vi "lv_icon.vi"(10 "Color icon in":T2, 11 "BW icon in":T2) -> (0 "Error code out":i32=43, 2 "Color icon out":T2, 3 "BW icon out":T2)   [LabVIEW 2021, in "lv_icon.lvlib"]
doc: "<p>Display this dialog box in one of the following ways:</p>\n\n<ul>\n<li>Double-click the <a href=\"nihelplauncher://docs/csh?context=lvcore_lvconcepts_using_icons\">icon</a> in the upper right corner of the front panel window, block diagram window, or <a href=\"nihelplauncher://docs/csh?context=lvcore_lvconcepts_custom_cont_ind_type\">Control Editor</a> window.</li>\n<li>Right-click the icon in the upper right corner of the front panel window, block diagram window, or <strong>Control Editor</strong> window and select <strong>Edit Icon</strong> from the shortcut menu.</li>\n<li>Select <strong>File<span class=\"U+187\">>></span>VI Properties</strong> or <strong>File<span class=\"U+187\">>></span>Control Properties</strong> to display the <a href=\"nihelplauncher://docs/csh?context=lvcore_lvdialog_vi_properties_dialog_box\">VI Properties</a> dialog box or <strong>Control Properties</strong> dialog box, respectively. Then select <strong>General</strong> from the <strong>Category</strong> pull-down menu and click the <strong>Edit Icon</strong> button.</li>\n<li>Right-click a project library, statechart, class, or XControl item in the <a href=\"nihelplauncher://docs/csh?context=lvcore_lvconcepts_using_labview_projects\">Project Explorer</a> window and select <strong> Properties</strong> from the shortcut menu to display the corresponding <strong>Properties</strong> dialog box. Then click the <strong>Edit</strong> button on the <strong>General Settings</strong> page.</li>\n</ul>\n\n<p>Use this dialog box to <a href=\"nihelplauncher://docs/csh?context=lvcore_lvhowto_creating_icons\">create and edit icons</a>.</p>"
uses:
  <vilib>/LabVIEW Icon API/lv_icon/lv_icon.lvlib
  <vilib>/LabVIEW Icon API/lv_icon/Controls/BodyText.ctl
  <vilib>/LabVIEW Icon API/lv_icon/Controls/Font.ctl
  <vilib>/LabVIEW Icon API/lv_icon/Controls/Alignment.ctl
  <vilib>/LabVIEW Icon API/lv_icon/Controls/Layer.ctl
  <resource>/plugins/NIIconEditor/Controls/LayerList.ctl
  <resource>/plugins/NIIconEditor/Controls/NewLayer.ctl
  <resource>/plugins/NIIconEditor/Controls/DeleteLayer.ctl
  <resource>/plugins/NIIconEditor/Controls/Arrow Up.ctl
  <resource>/plugins/NIIconEditor/Controls/Arrow Down.ctl
  <resource>/plugins/NIIconEditor/Controls/Framework Templates.ctl
  <vilib>/LabVIEW Icon API/lv_icon/Controls/Graphic.ctl
  <resource>/plugins/NIIconEditor/Controls/ColorChange.ctl
  <vilib>/LabVIEW Icon API/lv_icon/Controls/IEColor.ctl
  <resource>/plugins/NIIconEditor/Controls/Rotate.ctl
  <resource>/plugins/NIIconEditor/Controls/Flip.ctl
  <resource>/plugins/NIIconEditor/Controls/Tools.ctl
  <resource>/plugins/NIIconEditor/Controls/Pen.ctl
  <resource>/plugins/NIIconEditor/Controls/Line.ctl
  <resource>/plugins/NIIconEditor/Controls/Dropper.ctl
  <resource>/plugins/NIIconEditor/Controls/Fill.ctl
  <resource>/plugins/NIIconEditor/Controls/IERect.ctl
  <resource>/plugins/NIIconEditor/Controls/FRect.ctl
  <resource>/plugins/NIIconEditor/Controls/Circle.ctl
  <resource>/plugins/NIIconEditor/Controls/FCircle.ctl
  <resource>/plugins/NIIconEditor/Controls/Rubber.ctl
  <resource>/plugins/NIIconEditor/Controls/Text.ctl
  <resource>/plugins/NIIconEditor/Controls/Selection.ctl
  <resource>/plugins/NIIconEditor/Controls/Move.ctl
  <resource>/plugins/NIIconEditor/Controls/TextMarker.ctl
  <vilib>/picture/picture.llb/imagedata.ctl
  <resource>/plugins/NIIconEditor/Controls/Refresh.ctl
  <resource>/plugins/NIIconEditor/Controls/References Cluster.ctl
  <vilib>/Utility/miscctls.llb/LVPoint32TypeDef.ctl
  <vilib>/LabVIEW Icon API/lv_icon/Controls/Pathes.ctl
  <resource>/plugins/NIIconEditor/Controls/Path&Icon.ctl
  <resource>/plugins/NIIconEditor/Class/Ants/Ants.lvclass
  <resource>/plugins/NIIconEditor/Class/FakedArray/FakedArray.lvclass
  <vilib>/LabVIEW Icon API/lv_icon/Classes/Icon/Icon.lvclass
  <resource>/plugins/NIIconEditor/Class/Icon Library/Glyph.lvclass
panel:
  out "LabVIEW Icon out":string
  in  "LabVIEW Icon in":string
  out "Terminals":picture
  out "Preview2":picture
  out "TextMarker":T1="^"
  in  "Help":bool
  in  "Cancel":bool
  in  "OK":bool
  out "XYZ":string="X: 14\nY: 31\nZ: 1"
  out "RGB":string="R: 0\nG: 0\nB: 0"
  out "Icon":picture
  out "Clipboard":picture
  in  "Tab Control":T3(tab)
  in  "refreshTemplates":T4
  out "templates path str":string
  in  "Templates":string(tree)="<All>"
  in  "Filter templates by keyword":string
  in  "Framework Templates":T5={"Scrollbar"=0, "Path & Icon 1"={"Rectangle"={"left"=0, "top"=0, "right"=32, "bottom"=32}, "Path"=path "C:/Users/tsandris/Documents/LabVIEW Data/Icon Templates/VI/Frameworks/_blank.png", "Image"=bytes[0], "Filter"="VI\\Frameworks", "FileName"="_blank"}, "Path & Icon 2"={"Rectangle"={"left"=0, "top"=0, "right"=32, "bottom"=32}, "Path"=path "C:/Users/tsandris/Documents/LabVIEW Data/Icon Templates/Library/Frameworks/_blank.png", "Image"=bytes[0], "Filter"="Library\\Frameworks", "FileName"="_blank"}, "Path & Icon 3"={"Rectangle"={"left"=0, "top"=0, "right"=0, "bottom"=0}, "Path"=path "", "Image"=bytes[0], "Filter"="", "FileName"=""}, "Path & Icon 4"={"Rectangle"={"left"=0, "top"=0, "right"=0, "bottom"=0}, "Path"=path "", "Image"=bytes[0], "Filter"="", "FileName"=""}, "Path & Icon 5"={"Rectangle"={"left"=0, "top"=0, "right"=0, "bottom"=0}, "Path"=path "", "Image"=bytes[0], "Filter"="", "FileName"=""}, "Path & Icon 6"={"Rectangle"={"left"=0, "top"=0, "right"=0, "bottom"=0}, "Path"=path "", "Image"=bytes[0], "Filter"="", "FileName"=""}, "Path & Icon 7"={"Rectangle"={"left"=0, "top"=0, "right"=0, "bottom"=0}, "Path"=path "", "Image"=bytes[0], "Filter"="", "FileName"=""}, "Path & Icon 8"={"Rectangle"={"left"=0, "top"=0, "right"=0, "bottom"=0}, "Path"=path "", "Image"=bytes[0], "Filter"="", "FileName"=""}, "Path & Icon 9"={"Rectangle"={"left"=0, "top"=0, "right"=0, "bottom"=0}, "Path"=path "", "Image"=bytes[0], "Filter"="", "FileName"=""}, "Path & Icon 10"={"Rectangle"={"left"=0, "top"=0, "right"=0, "bottom"=0}, "Path"=path "", "Image"=bytes[0], "Filter"="", "FileName"=""}, "Path & Icon 11"={"Rectangle"={"left"=0, "top"=0, "right"=0, "bottom"=0}, "Path"=path "", "Image"=bytes[0], "Filter"="", "FileName"=""}, "Path & Icon 12"={"Rectangle"={"left"=0, "top"=0, "right"=0, "bottom"=0}, "Path"=path "", "Image"=bytes[0], "Filter"="", "FileName"=""}, "Path & Icon 13"={"Rectangle"={"left"=0, "top"=0, "right"=0, "bottom"=0}, "Path"=path "", "Image"=bytes[0], "Filter"="", "FileName"=""}, "Path & Icon 14"={"Rectangle"={"left"=0, "top"=0, "right"=0, "bottom"=0}, "Path"=path "", "Image"=bytes[0], "Filter"="", "FileName"=""}, "Path & Icon 15"={"Rectangle"={"left"=0, "top"=0, "right"=0, "bottom"=0}, "Path"=path "", "Image"=bytes[0], "Filter"="", "FileName"=""}, "Path & Icon 16"={"Rectangle"={"left"=0, "top"=0, "right"=0, "bottom"=0}, "Path"=path "", "Image"=bytes[0], "Filter"="", "FileName"=""}, "Path & Icon 17"={"Rectangle"={"left"=0, "top"=0, "right"=0, "bottom"=0}, "Path"=path "", "Image"=bytes[0], "Filter"="", "FileName"=""}, "Path & Icon 18"={"Rectangle"={"left"=0, "top"=0, "right"=0, "bottom"=0}, "Path"=path "", "Image"=bytes[0], "Filter"="", "FileName"=""}, "Path & Icon 19"={"Rectangle"={"left"=0, "top"=0, "right"=0, "bottom"=0}, "Path"=path "", "Image"=bytes[0], "Filter"="", "FileName"=""}, "Path & Icon 20"={"Rectangle"={"left"=0, "top"=0, "right"=0, "bottom"=0}, "Path"=path "", "Image"=bytes[0], "Filter"="", "FileName"=""}, "Path & Icon 21"={"Rectangle"={"left"=0, "top"=0, "right"=0, "bottom"=0}, "Path"=path "", "Image"=bytes[0], "Filter"="", "FileName"=""}, "Path & Icon 22"={"Rectangle"={"left"=0, "top"=0, "right"=0, "bottom"=0}, "Path"=path "", "Image"=bytes[0], "Filter"="", "FileName"=""}, "Path & Icon 23"={"Rectangle"={"left"=0, "top"=0, "right"=0, "bottom"=0}, "Path"=path "", "Image"=bytes[0], "Filter"="", "FileName"=""}, "Path & Icon 24"={"Rectangle"={"left"=0, "top"=0, "right"=0, "bottom"=0}, "Path"=path "", "Image"=bytes[0], "Filter"="", "FileName"=""}, "Path & Icon 25"={"Rectangle"={"left"=0, "top"=0, "right"=0, "bottom"=0}, "Path"=path "", "Image"=bytes[0], "Filter"="", "FileName"=""}, "Path & Icon 26"={"Rectangle"={"left"=0, "top"=0, "right"=0, "bottom"=0}, "Path"=path "", "Image"=bytes[0], "Filter"="", "FileName"=""}, "Path & Icon 27"={"Rectangle"={"left"=0, "top"=0, "right"=0, "bottom"=0}, "Path"=path "", "Image"=bytes[0], "Filter"="", "FileName"=""}, "Path & Icon 28"={"Rectangle"={"left"=0, "top"=0, "right"=0, "bottom"=0}, "Path"=path "", "Image"=bytes[0], "Filter"="", "FileName"=""}, "Path & Icon 29"={"Rectangle"={"left"=0, "top"=0, "right"=0, "bottom"=0}, "Path"=path "", "Image"=bytes[0], "Filter"="", "FileName"=""}, "Path & Icon 30"={"Rectangle"={"left"=0, "top"=0, "right"=0, "bottom"=0}, "Path"=path "", "Image"=bytes[0], "Filter"="", "FileName"=""}}
  in  "Body Text":T7={"Line 1 text"="", "Line 2 text"="", "Line 3 text"="", "Line 4 text"="", "Line 1 color"=0, "Line 2 color"=0, "Line 3 color"=0, "Line 4 color"=0, "Body Text Spec"={"Font"="", "Alignment"=1, "Size"=9}, "Center text vertically"=TRUE, "Capitalize Text"=TRUE} {"Body Text Spec"."Alignment" items=["left", "center", "right"]}
  in  "Filter glyphs by keyword":string
  in  "Glyphs":string(tree)="<All>"
  out "glyph path str":string
  out "Glyphs []":T6[][](array[typedef])
  in  "refreshGlyphs":T4
  in  "Add Layer":T10
  in  "Remove Layer":T11
  in  "Move Down":T12
  in  "Move Up":T13
  in  "Icon Template":T14={"LayerIcon"=bytes[0], "LayerName"="", "Opacity"=100, "Visibility?"=TRUE} {"Opacity" scale=0.0..100.0}
  in  "Icon Text":T14={"LayerIcon"=bytes[0], "LayerName"="Icon Text", "Opacity"=100, "Visibility?"=TRUE} {"Opacity" scale=0.0..100.0}
  in  "User Layers":T15={"Scrollbar"=0, "Layer 1"={"LayerIcon"=bytes[0], "LayerName"="VI Icon", "Opacity"=100, "Visibility?"=TRUE}, "Layer 2"={"LayerIcon"=bytes[3230], "LayerName"="", "Opacity"=100, "Visibility?"=TRUE}, "Layer 3"={"LayerIcon"=bytes[3230], "LayerName"="", "Opacity"=100, "Visibility?"=TRUE}, "Layer 4"={"LayerIcon"=bytes[3230], "LayerName"="", "Opacity"=100, "Visibility?"=TRUE}} {"Layer 4"."Opacity" scale=0.0..100.0; "Layer 3"."Opacity" scale=0.0..100.0; "Layer 2"."Opacity" scale=0.0..100.0; "Layer 1"."Opacity" scale=0.0..100.0}
  out "Preview":picture
  in  "Horizontal Flip":T16
  in  "Clockwise Rotate":T17
  in  "Swap":T18
  in  "Line Color":T19
  in  "Fill Color":T19=16777215
  in  "Tools":T20=enum."Rectangle"
  # "Clipboard control. Anything made on this\ncontrol will show up in the clipboard image data."
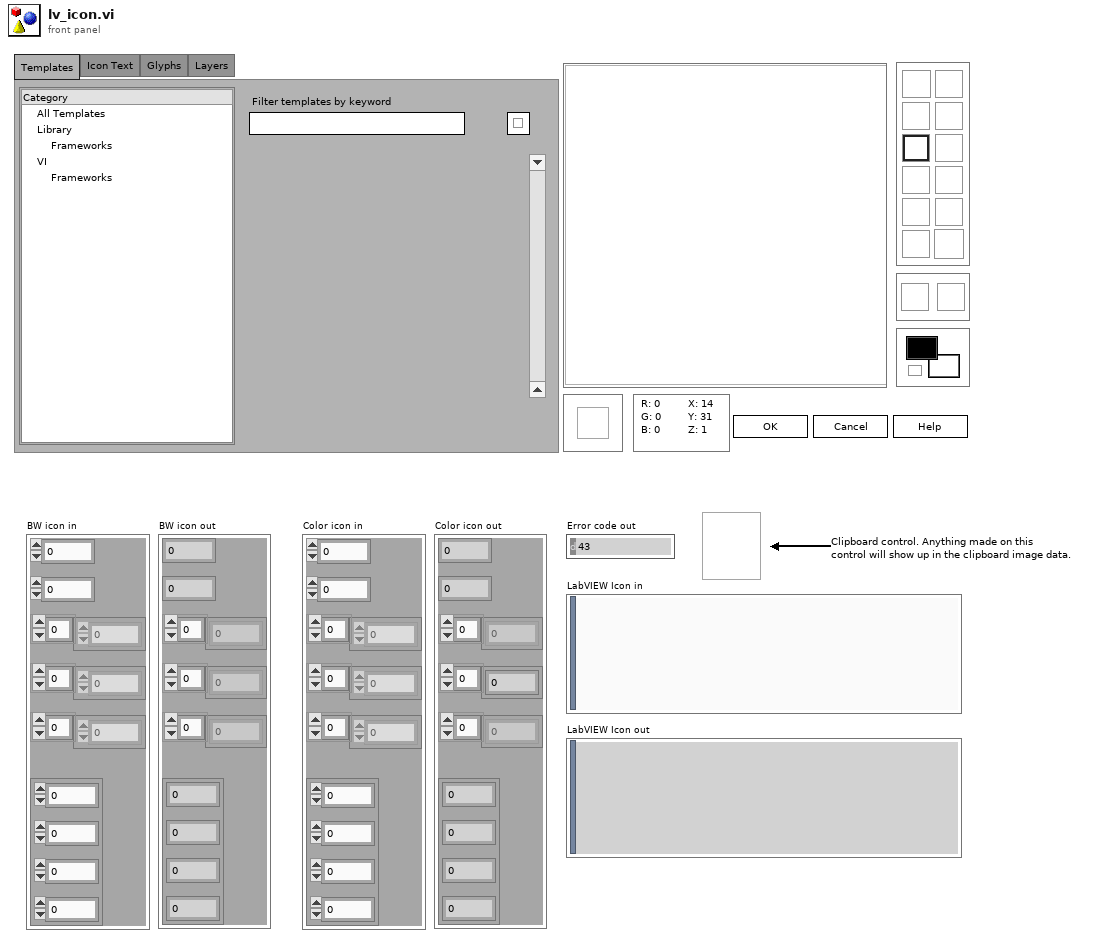
[diagram p1: front panel]
types:
  T1 = typedef "TextMarker.ctl" = string
  T2 = typedef "imagedata.ctl" = cluster{"image type":i32, "image depth":i32, "image":u8[], "mask":u8[], "colors":u32[], "Rectangle":cluster{"left":i16, "top":i16, "right":i16, "bottom":i16}}
  T3 = enum32{"Templates", "Icon Text", "Glyphs", "Layers"}
  T4 = typedef "Refresh.ctl" = bool
  T5 = typedef "Framework Templates.ctl" = cluster{"Scrollbar":i32, "Path & Icon 1":T6, "Path & Icon 2":T6, "Path & Icon 3":T6, "Path & Icon 4":T6, "Path & Icon 5":T6, "Path & Icon 6":T6, "Path & Icon 7":T6, "Path & Icon 8":T6, "Path & Icon 9":T6, "Path & Icon 10":T6, "Path & Icon 11":T6, "Path & Icon 12":T6, "Path & Icon 13":T6, "Path & Icon 14":T6, "Path & Icon 15":T6, "Path & Icon 16":T6, "Path & Icon 17":T6, "Path & Icon 18":T6, "Path & Icon 19":T6, "Path & Icon 20":T6, "Path & Icon 21":T6, "Path & Icon 22":T6, "Path & Icon 23":T6, "Path & Icon 24":T6, "Path & Icon 25":T6, "Path & Icon 26":T6, "Path & Icon 27":T6, "Path & Icon 28":T6, "Path & Icon 29":T6, "Path & Icon 30":T6}
  T6 = typedef "Graphic.ctl" = cluster{"Rectangle":cluster{"left":i16, "top":i16, "right":i16, "bottom":i16}, "Path":path, "Image":picture, "Filter":string, "FileName":string}
  T7 = typedef "BodyText.ctl" = cluster{"Line 1 text":string, "Line 2 text":string, "Line 3 text":string, "Line 4 text":string, "Line 1 color":u32, "Line 2 color":u32, "Line 3 color":u32, "Line 4 color":u32, "Body Text Spec":cluster{"Font":T8, "Alignment":T9, "Size":u8}, "Center text vertically":bool, "Capitalize Text":bool}
  T8 = typedef "Font.ctl" = string
  T9 = typedef "Alignment.ctl" = u16
  T10 = typedef "NewLayer.ctl" = bool
  T11 = typedef "DeleteLayer.ctl" = bool
  T12 = typedef "Arrow Down.ctl" = bool
  T13 = typedef "Arrow Up.ctl" = bool
  T14 = typedef "Layer.ctl" = cluster{"LayerIcon":picture, "LayerName":string, "Opacity":u8, "Visibility?":bool}
  T15 = typedef "LayerList.ctl" = cluster{"Scrollbar":i32, "Layer 1":T14, "Layer 2":T14, "Layer 3":T14, "Layer 4":T14}
  T16 = typedef "Flip.ctl" = bool
  T17 = typedef "Rotate.ctl" = bool
  T18 = typedef "ColorChange.ctl" = bool
  T19 = typedef "IEColor.ctl" = u32
  T20 = typedef "Tools.ctl" = enum32{"Pencil", "Line", "Dropper", "Fill", "Rectangle", "Filled Rectangle", "Ellipse", "Filled Ellipse", "Eraser", "Text", "Select", "Move"}
  T21 = enum32{"Invalid", "Standard", "Closed", "Hidden", "Minimized", "Maximized"}
  T22 = typedef "lv_icon.lvlib/References Cluster.ctl" = cluster{"Add Layer":refnum<vi>, "Remove Layer":refnum<vi>, "Line Text":refnum<vi>[], "Body Text Spec":refnum<vi>, "DNL_Font":refnum<vi>, "glyph path str":refnum<vi>, "templates path str":refnum<vi>, "Arrow Up":refnum<vi>, "Arrow Down":refnum<vi>, "IE VI Ref":refnum<vi>, "Glyphs tree":refnum<vi>, "Templates tree":refnum<vi>, "Layer Icon Text":refnum<vi>, "Layer Template":refnum<vi>, "Body Text":refnum<vi>, "Search Templates":refnum<vi>, "TextMarker":refnum<vi>, "Tab Control":refnum<vi>, "Search Glyphs":refnum<vi>, "Line Color":refnum<vi>, "DNL_Glyphs []":refnum<vi>, "Fill Color":refnum<vi>, "Tools":refnum<vi>, "Icon":refnum<vi>, "Preview":refnum<vi>, "Ants":refnum<vi>, "Terminals":refnum<vi>, "menu reference":refnum<k9>, "LayerNames":refnum<vi>[], "GlyphLoadAnimation":refnum<vi>, "TemplateLoadAnimation":refnum<vi>, "refreshGlyphs":refnum<vi>, "refreshTemplates":refnum<vi>}
  T23 = cluster{"Global stop?":refnum<user-event>, "Templates":refnum<user-event>, "Glyphs":refnum<user-event>}
  T24 = typedef "lv_icon.lvlib/Global Data.ctl" = cluster{"Class":T25, "Ref":T22, "Support":T26}
  T25 = typedef "IE Classes.ctl" = cluster{"Ants":refnum<class "Ants.lvclass">, "Layer":refnum<class "FakedArray.lvclass">, "Templates":refnum<class "FakedArray.lvclass">, "Icon":refnum<class "Icon.lvclass">, "Glyph":refnum<class "Glyph.lvclass">, "Settings":refnum<class "Settings.lvclass">, "Tools":refnum<class "Tools Paint.lvclass">}
  T26 = typedef "SupportClass.ctl" = cluster{"AntsRect":cluster{"left":i16, "top":i16, "right":i16, "bottom":i16}, "Mouse Move Coords":T27, "Mouse Down Coords":T27, "Temp Coord":T27, "Action":T28, "Edge Color":T19, "Fill Color":T19, "Mouse Down?":bool, "Draft Mode?":bool, "Temp Icon":picture, "CTRL Pressed":bool, "Move Selection?":bool, "AntsRect Orig":cluster{"left":i16, "top":i16, "right":i16, "bottom":i16}, "Text":string, "TM Set?":bool, "Mouse inside icon?":bool, "Tool (old value)":u32, "Pencil Move Color":u32, "Swap Colors?":bool, "Shift pressed?":bool}
  T27 = typedef "LVPoint32TypeDef.ctl" = cluster{"Horizontal":i32, "Vertical":i32}
  T28 = typedef "SupportClass_Action.ctl" = enum16{"Default", "Move Selection", "Glyph Library", "Tool"}
  T29 = typedef "Pathes.ctl" = enum16{"Root Path", "Icon Templates", "Icon Templates VI", "Icon Templates Lib", "Glyphs"}
  T30 = typedef "Path&Icon.ctl" = cluster{"Rectangle":cluster{"left":i16, "top":i16, "right":i16, "bottom":i16}, "Path":path, "Image":picture, "Filter":string, "FileName":string}
  T31 = typedef "lveventtype.ctl" = enum32{"Null", "Timeout", "Annotation Menu Selection", "Annotation Menu Selection?", "App Instance Close", "App Instance Close?", "Autoscale Range Change", "Bookmark Info Change", "Cell Edit", "Cell Edit?", "Cursor Grab", "Cursor Grab?", "Cursor Menu Selection", "Cursor Menu Selection?", "Cursor Move", "Cursor Release", "Data Change", "Direction Change", "Display State Change", "Drag Ended", "Drag Enter", "Drag Leave", "Drag Over", "Drag Source Update", "Drag Starting", "Drag Starting?", "Drop", "Exec State Change", "Key Down", "Key Down?", "Key Repeat", "Key Repeat?", "Key Up", "Listbox Double Click", "Menu Activation?", "Menu Selection (App)", "Menu Selection? (App)", "Menu Selection (User)", "Mouse Down", "Mouse Down?", "Mouse Enter", "Mouse Leave", "Mouse Move", "Mouse Up", "Mouse Wheel", "NI Security User Change (App)", "Pane Size", "Panel Close", "Panel Close?", "Panel Resize", "Plot Attribute Change", "Scale Range Change", "Shortcut Menu Activation?", "Shortcut Menu Selection (App)", "Shortcut Menu Selection? (App)", "Shortcut Menu Selection (User)", "Tree Double Click", "Tree Drag", "Tree Drag?", "Tree Drop", "Tree Drop?", "Tree Item Close", "Tree Item Close?", "Tree Item Open", "Tree Item Open?", "User Event", "Value Change"}
  T32 = typedef "eventvkey.ctl" = enum16{"ASCII", "Enter", "Return", "Shift", "Ctrl", "Alt", "Cmd", "Opt", "Caps", "NumLock", "Clear", "Break", "Up", "Down", "Left", "Right", "Insert", "Delete", "Home", "End", "PageUp", "PageDown", "Escape", "Help", "Pause", "ScrollLock", "F1", "F2", "F3", "F4", "F5", "F6", "F7", "F8", "F9", "F10", "F11", "F12", "F13", "F14", "F15", "F16", "F17", "F18", "F19", "F20", "F21", "F22", "F23", "F24", "Play", "VolumeUp", "VolumeDown", "Mute", "Two Byte Char"}
  T33 = cluster{"Shift":bool, "Ctrl":bool, "Alt":bool, "Cmd":bool, "Opt":bool}
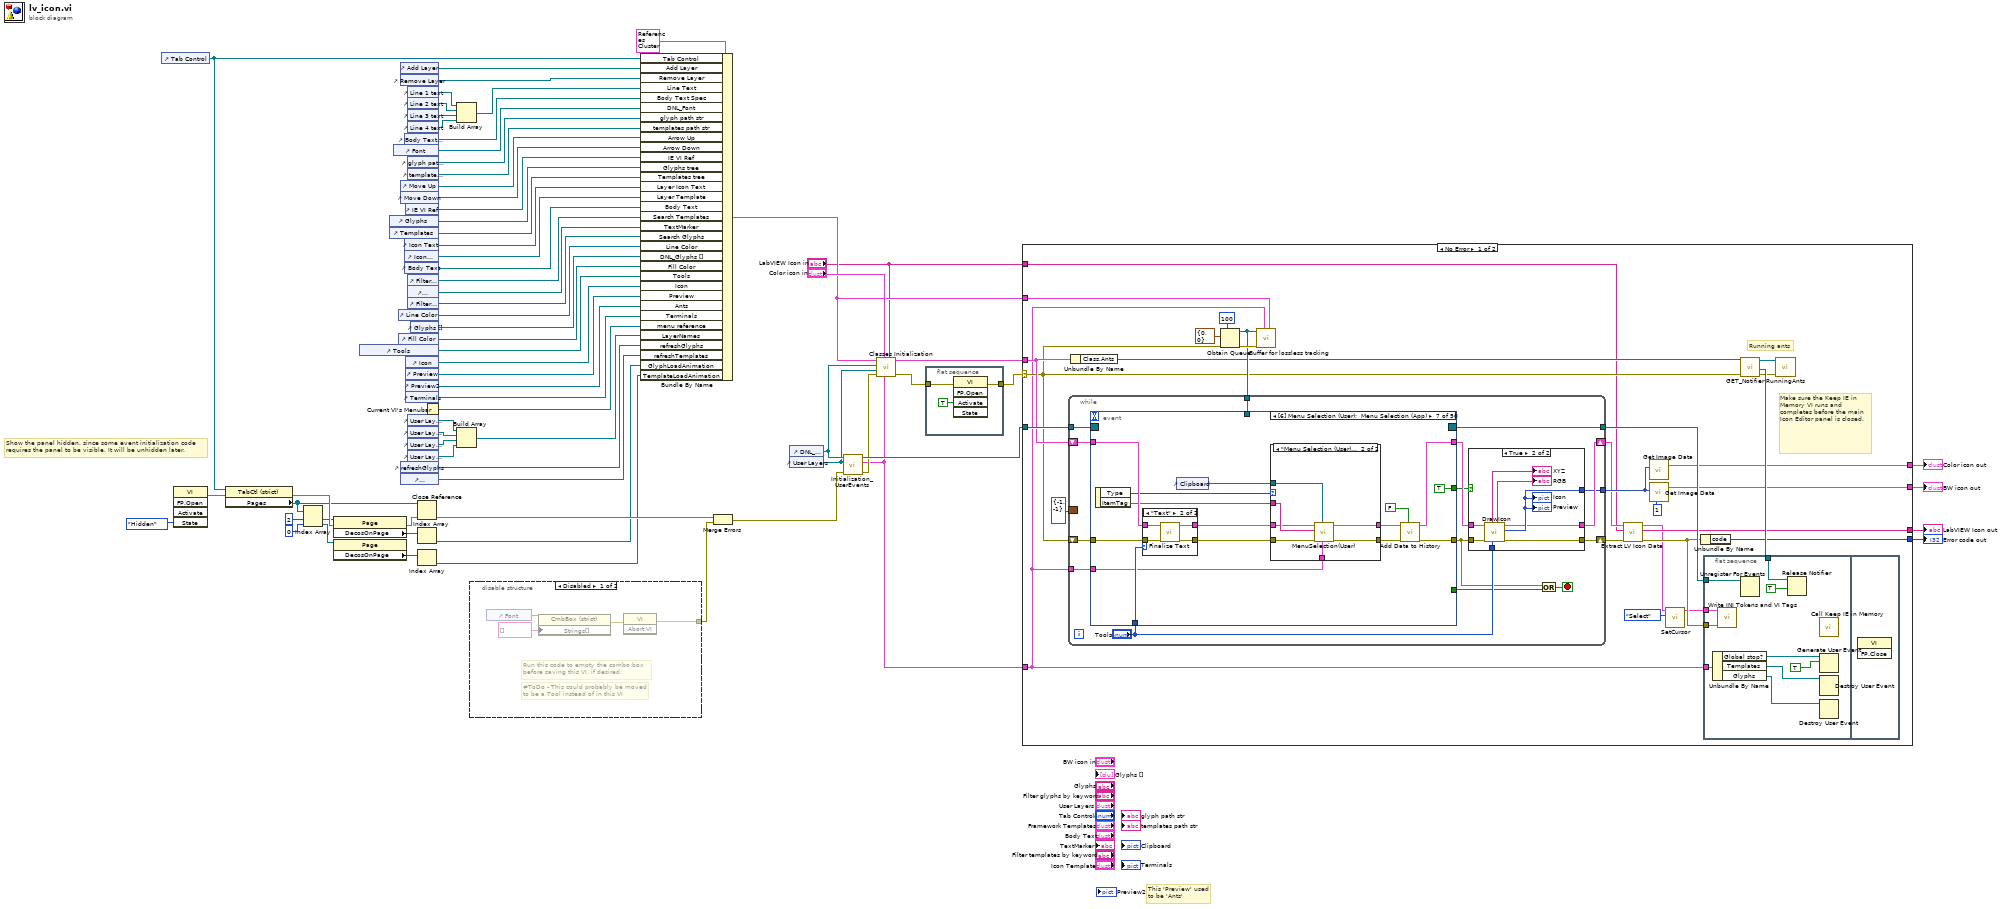
[diagram p0: block diagram]
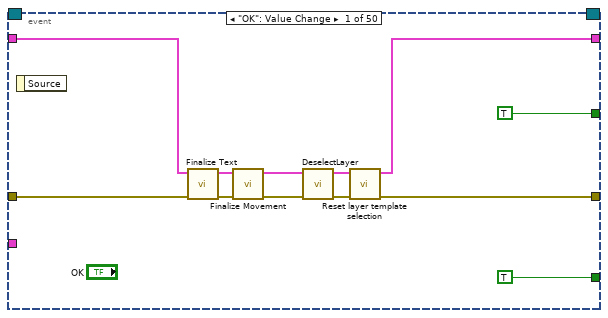
[diagram p4: hidden frame]
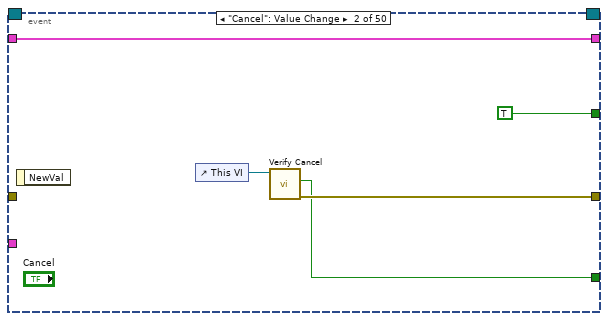
[diagram p5: hidden frame]
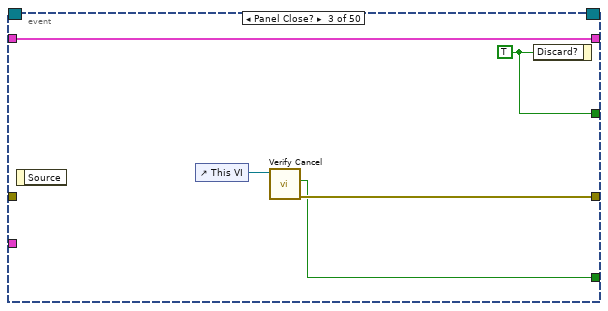
[diagram p6: hidden frame]
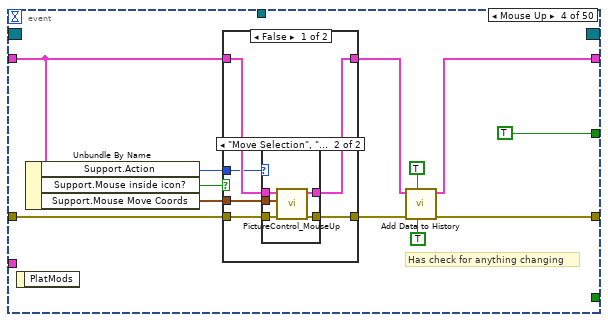
[diagram p7: hidden frame]
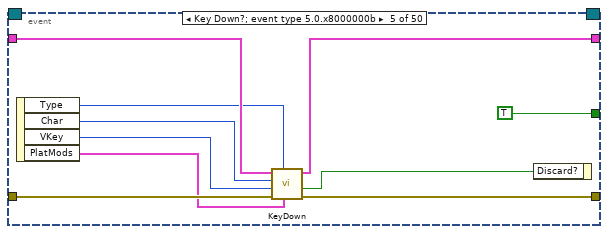
[diagram p10: hidden frame]
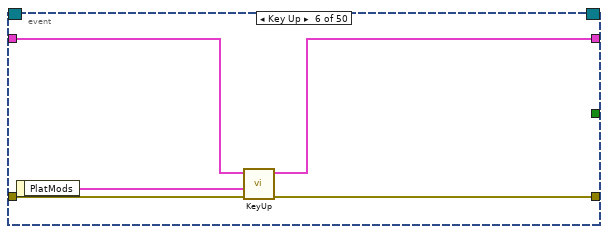
[diagram p11: hidden frame]
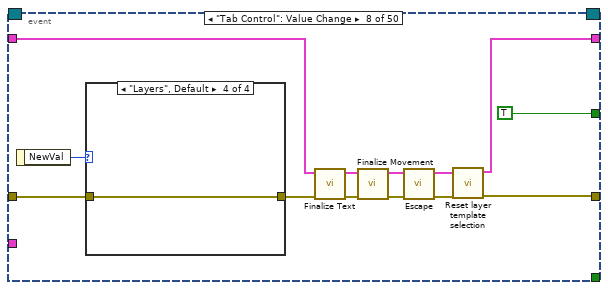
[diagram p14: hidden frame]
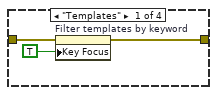
[diagram p15: hidden frame]
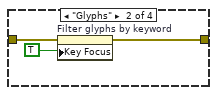
[diagram p16: hidden frame]
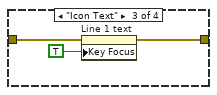
[diagram p17: hidden frame]
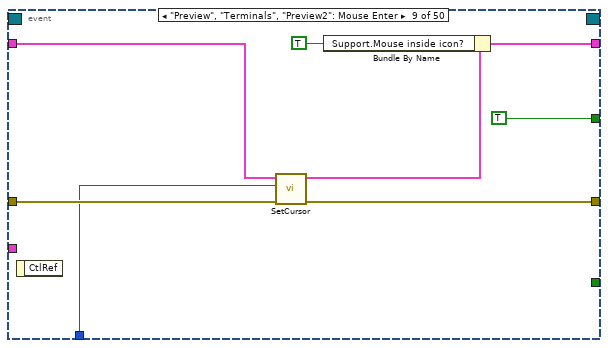
[diagram p18: hidden frame]
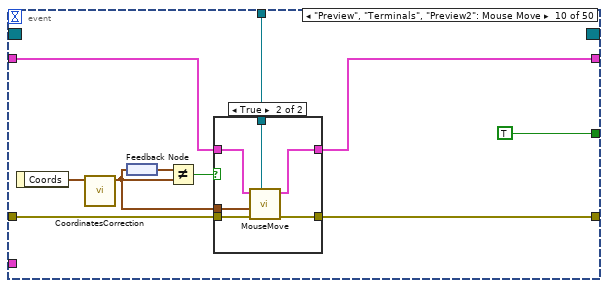
[diagram p19: hidden frame]
diagram:
  # "Show the panel hidden, since some event initialization code requires the panel to be visible. It will be unhidden later."
  # "This 'Preview' used\nto be 'Ants'"
  n1 = control-ref of="Tab Control"() -> (w4:refnum<vi>)
  n2 = invoke class="VI" method="FP.Open"("State"=T21."Hidden") -> (error out=w1:errorcluster)  [unwired: 4 in, 4 out]
  n3 = property class="TabCtl (strict)"(reference=w4, error in=w1) -> (error out=w14:errorcluster, "Pages"=w6:refnum<vi>[])  [unwired: 1 out]
  n4 = Index Array(array=w6, index #1=2 ("index"), index #2=0 ("index")) -> (element #1=w10:refnum<vi>, element #2=w11:refnum<vi>)
  n5 = property class="Page"(reference=w10, error in=w14) -> (error out=w7:errorcluster, "DecosOnPage"=w9:refnum<vi>[])  [unwired: 1 out]
  n6 = property class="Page"(reference=w11) -> ("DecosOnPage"=w8:refnum<vi>[])  [unwired: 1 in, 2 out]
  n7 = control-ref of="Tools"() -> (w68:refnum<vi>)
  n8 = control-ref of="Glyphs"() -> (w52:refnum<vi>)
  n9 = control-ref of="Templates"() -> (w53:refnum<vi>)
  n10 = control-ref of="Font"() -> (w34:refnum<vi>)
  n11 = control-ref of="Line Color"() -> (w66:refnum<vi>)
  n12 = control-ref of="Fill Color"() -> (w67:refnum<vi>)
  n13 = control-ref of="Add Layer"() -> (w37:refnum<vi>)
  n14 = control-ref of="Remove Layer"() -> (w38:refnum<vi>)
  n15 = control-ref of="Move Up"() -> (w49:refnum<vi>)
  n16 = control-ref of="Move Down"() -> (w50:refnum<vi>)
  n17 = control-ref of="refreshGlyphs"() -> (w24:refnum<vi>)
  n18 = control-ref of="refreshTemplates"() -> (w25:refnum<vi>)
  n19 = control-ref of="Body Text Spec"() -> (w46:refnum<vi>)
  n20 = control-ref of="Icon Text"() -> (w55:refnum<vi>)
  n21 = control-ref of="Icon Template"() -> (w56:refnum<vi>)
  n22 = control-ref of="Body Text"() -> (w61:refnum<vi>)
  n23 = control-ref of="IE VI Ref"() -> (w51:refnum<vi>)
  n24 = control-ref of="Icon"() -> (w69:refnum<vi>)
  n25 = control-ref of="Preview"() -> (w70:refnum<vi>)
  n26 = control-ref of="Preview2"() -> (w45:refnum<vi>)
  n27 = control-ref of="Terminals"() -> (w60:refnum<vi>)
  n28 = control-ref of="Line 1 text"() -> (w40:refnum<vi>)
  n29 = control-ref of="Line 2 text"() -> (w41:refnum<vi>)
  n30 = control-ref of="Line 3 text"() -> (w42:refnum<vi>)
  n31 = control-ref of="Line 4 text"() -> (w43:refnum<vi>)
  n32 = control-ref of="glyph path str"() -> (w47:refnum<vi>)
  n33 = control-ref of="templates path str"() -> (w48:refnum<vi>)
  n34 = control-ref of="Filter templates by keyword"() -> (w63:refnum<vi>)
  n35 = control-ref of="TextMarker"() -> (w64:refnum<vi>)
  n36 = control-ref of="Filter glyphs by keyword"() -> (w65:refnum<vi>)
  n37 = control-ref of="User Layer 1"() -> (w29:refnum<vi>)
  n38 = control-ref of="User Layer 2"() -> (w30:refnum<vi>)
  n39 = control-ref of="User Layer 3"() -> (w31:refnum<vi>)
  n40 = control-ref of="User Layer 4"() -> (w32:refnum<vi>)
  n41 = control-ref of="Glyphs []"() -> (w35:refnum<vi>)
  n42 = Close Reference(reference=w6, error in (no error)=w7) -> (error out=w5:errorcluster)
  n43 = Index Array(array=w9) -> (element=w3:refnum<vi>)  [unwired: 1 in]
  n44 = Index Array(array=w8) -> (element=w2:refnum<vi>)  [unwired: 1 in]
  n45 = Current VI's Menubar() -> (w59:refnum<k9>)
  n46 = Build Array(w40, w41, w42, w43) -> (w39:refnum<vi>[])
  n47 = Build Array(w29, w30, w31, w32) -> (w27:refnum<vi>[])
  n48 = disable-structure shown="Disabled" {
    disable-tunnel: [w72 _] -> w16
    frame Disabled {
      # "#ToDo - This could probably be moved\nto be a Tool instead of in this VI"
      # "Run this code to empty the combo box\nbefore saving this VI, if desired."
      n49 = control-ref of="Font"() -> (w75:refnum<vi>)
      n50 = property class="CmbBox (strict)"(reference=w75, "Strings[]"=string[] [] ("Strings []")) -> (error out=w73:errorcluster)  [unwired: 1 in, 1 out]
      n51 = invoke class="VI" method="Abort VI"(error in=w73) -> (error out=w72:errorcluster)  [unwired: 2 in, 2 out]
    }
    frame Enabled {
    }
  }
  n52 = Bundle By Name(cluster=T22 {"Add Layer"=refnum, "Remove Layer"=refnum, "Line Text"=[], "Body Text Spec"=refnum, "DNL_Font"=refnum, "glyph path str"=refnum, "templates path str"=refnum, "Arrow Up"=refnum, "Arrow Down"=refnum, "IE VI Ref"=refnum, "Glyphs tree"=refnum, "Templates tree"=refnum, "Layer Icon Text"=refnum, "Layer Template"=refnum, "Body Text"=refnum, "Search Templates"=refnum, "TextMarker"=refnum, "Tab Control"=refnum, "Search Glyphs"=refnum, "Line Color"=refnum, "DNL_Glyphs []"=refnum, "Fill Color"=refnum, "Tools"=refnum, "Icon"=refnum, "Preview"=refnum, "Ants"=refnum, "Terminals"=refnum, "menu reference"=refnum, "LayerNames"=[], "GlyphLoadAnimation"=refnum, "TemplateLoadAnimation"=refnum, "refreshGlyphs"=refnum, "refreshTemplates"=refnum} ("references"), "Tab Control"=w4, "Add Layer"=w37, "Remove Layer"=w38, "Line Text"=w39, "Body Text Spec"=w46, "DNL_Font"=w34, "glyph path str"=w47, "templates path str"=w48, "Arrow Up"=w49, "Arrow Down"=w50, "IE VI Ref"=w51, "Glyphs tree"=w52, "Templates tree"=w53, "Layer Icon Text"=w55, "Layer Template"=w56, "Body Text"=w61, "Search Templates"=w63, "TextMarker"=w64, "Search Glyphs"=w65, "Line Color"=w66, "DNL_Glyphs []"=w35, "Fill Color"=w67, "Tools"=w68, "Icon"=w69, "Preview"=w70, "Ants"=w45, "Terminals"=w60, "menu reference"=w59, "LayerNames"=w27, "refreshGlyphs"=w24, "refreshTemplates"=w25, "GlyphLoadAnimation"=w3, "TemplateLoadAnimation"=w2) -> (w28:T22)
  n53 = Merge Errors(w5, w16) -> (w15:errorcluster)
  n54 = control-ref of="DNL_Framework Templates"() -> (w18:refnum<vi>)
  n55 = control-ref of="User Layers"() -> (w17:refnum<vi>)
  n56 = call <resource>:"Initialization_UserEvents.vi"("error in"=w15, "Layer Clusters"=w17, "DNL_Framework Templates"=w18) -> ("error out"=w57:errorcluster, "User events"=w19:T23, "Events"=w62:refnum<event-registration>)  [unwired: 6 out]
  n57 = call <resource>:"Classes Initialization.vi"("LabVIEW Icon in"="LabVIEW Icon in", "User events"=w19, "Color icon in"="Color icon in", "error in"=w57, "Layer Clusters"=w17, "DNL_Framework Templates"=w18, "Ref Cluster"=w28) -> ("error out"=w21:errorcluster, "Data out"=w44:T24)  [unwired: 3 out]
  n58 = flat-sequence {
    tunnel: w21 -> [w77]
    tunnel: [w76] -> w20
    frame #0 {
      n59 = invoke class="VI" method="FP.Open"(error in=w77, "Activate"=TRUE ("Activate?")) -> (error out=w76:errorcluster)  [unwired: 3 in, 4 out]
    }
  }
  n60 = case shown="No Error" w20 {
    selector: w20 -> [w88 w777]
    tunnel: w62 -> [w105 _]
    tunnel: [w103 w778] -> w58
    tunnel: [w100 _] -> w54
    tunnel: w19 -> [w79 _]
    tunnel: w44 -> [w93 _]
    tunnel: w28 -> [w91 _]
    tunnel: [w90 _] -> w36
    tunnel: "LabVIEW Icon in" -> [w83 w776]
    tunnel: [w86 w776] -> w33
    frame No Error {
      # "Make sure the Keep IE in Memory VI runs and completes before the main Icon Editor panel is closed."
      # "Running ants"
      n61 = Unbundle By Name(w93) -> ("Class.Ants"=w92:refnum<class "Ants.lvclass">)
      n62 = Obtain Queue(max queue size (-1, unlimited)=100, element data type=T27 {"Horizontal"=0, "Vertical"=0} ("Coords"), error in (no error)=w88) -> (queue out=w94:refnum<queue>, error out=w95:errorcluster)  [unwired: 1 in, 2 out]
      n63 = while {
        shift-right: [w111] -> w85
        shift-left: w88 -> [w118]
        tunnel: [w115] -> w106
        tunnel: w105 -> [w114]
        tunnel: [w113] -> w102
        tunnel: w94 -> [w109]
        shift-right: [w120] -> w87
        shift-left: w93 -> [w108]
        border: T27 {"Horizontal"=-1, "Vertical"=-1} ("Corrected Out") -> [_]
        tunnel: w79 -> [w107]
        stop <- w116 stop-if-true
        n64 = event shown="[6] Menu Selection (User);  Menu Selection (App)" {
          selector: w114 -> [_ _ _ _ _ _ _ _ _ _ _ _ _ _ _ _ _ _ _ _ _ _ _ _ _ _ _ _ _ _ _ _ _ _ _ _ _ _ _ _ _ _ _ _ _ _ _ _ _ _]
          dyn-events: [_ _ _ _ _ _ _ _ _ _ _ _ _ _ _ _ _ _ _ _ _ _ _ _ _ _ _ _ _ _ _ _ _ _ _ _ _ _ _ _ _ _ _ _ _ _ _ _ _ _] -> w115
          timeout: _ -> [_ _ _ _ _ _ _ _ _ _ _ _ _ _ _ _ _ _ _ _ _ _ _ _ _ _ _ _ _ _ _ _ _ _ _ _ _ _ _ _ _ _ _ _ _ _ _ _ _ _]
          tunnel: [w137 w147 w152 w157 w189 w195 w199 w234 w255 w265 w278 w295 w299 w305 w309 w322 w334 w348 w363 w374 w399 w406 w417 w433 w454 w462 w480 w500 w505 w509 w516 w527 w547 w562 w577 w588 w601 w617 w626 w635 w658 w671 w686 w696 w698 w717 w734 w754 w761 w763] -> w112
          tunnel: w118 -> [w139 _ _ w163 w190 w194 w207 w236 w256 w266 w278 w296 w302 w307 w314 w326 w333 w342 w365 w383 w400 w409 w422 w435 w457 w476 w488 w501 w506 w510 w517 w539 w552 w565 w581 w589 w607 w621 w627 w638 w661 w679 w689 w695 w707 w724 w738 w755 w761 w764]
          tunnel: [TRUE w146 w151 _ _ _ _ _ _ _ _ _ _ _ _ _ _ _ _ _ _ _ _ _ _ _ _ _ _ _ _ _ _ _ _ _ _ _ _ _ _ _ _ _ _ _ _ _ _ _] -> w117
          tunnel: "Tools" -> [_ _ _ _ _ _ w205 _ w254 _ _ _ _ _ _ _ _ _ _ _ _ _ _ _ _ _ _ _ _ _ _ _ _ _ _ _ _ _ _ _ _ _ _ _ _ _ _ _ _ _]
          tunnel: [TRUE TRUE ("Yes") w150 TRUE ("Yes") TRUE _ TRUE TRUE TRUE TRUE _ TRUE TRUE _ TRUE TRUE TRUE TRUE TRUE TRUE _ _ TRUE TRUE _ _ _ _ _ _ TRUE TRUE TRUE _ TRUE _ TRUE _ _ TRUE TRUE _ _ _ _ _ TRUE _ _ _] -> w110
          tunnel: w109 -> [_ _ _ _ _ _ _ _ _ w263 _ _ _ _ _ _ _ _ _ _ _ _ _ _ _ _ _ _ _ _ _ _ _ _ _ _ _ _ _ _ _ _ _ _ _ _ _ _ _ _]
          tunnel: w108 -> [w136 w148 w153 w162 w185 w193 w210 w232 w252 w262 w275 w292 w298 w304 w313 w325 w332 w344 w358 w370 w403 w405 w413 w431 w450 w467 w485 w498 w508 w512 w514 w535 w543 w560 w573 w586 w599 w623 w624 w645 w656 w669 w685 w693 w703 w722 w731 w752 w760 w765]
          tunnel: [w132 w148 w153 w155 w182 w191 w201 w226 w250 w261 w277 w291 w297 w303 w318 w320 w330 w347 w359 w375 w388 w404 w411 w429 w449 w460 w481 w498 w508 w511 w513 w528 w541 w559 w572 w585 w598 w615 w625 w631 w655 w673 w684 w691 w699 w716 w728 w752 w760 w765] -> w121
          tunnel: w107 -> [_ _ _ _ _ _ w197 _ _ _ _ _ _ _ _ _ _ _ _ _ _ _ _ _ _ _ _ w499 _ _ _ _ _ _ _ _ _ _ _ _ _ _ _ _ _ _ _ w753 _ _]
          event "OK": Value Change {
            n65 = event-data() -> ()  [unwired: 2 out]
            n66 = call <resource>:"Finalize Text.vi"("error in (no error)"=w139, "Data in"=w136) -> ("error out"=w140:errorcluster, "Data out"=w135:T24)  [unwired: 8 out]
            n67 = call <resource>:"Finalize Movement.vi"("error in (no error)"=w140, "Data in"=w135) -> ("error out"=w141:errorcluster, "Data out"=w134:T24)  [unwired: 1 in, 7 out]
            n68 = call <resource>:"DeselectLayer.vi"("error in (no error)"=w141, "Data in"=w134) -> ("error out"=w138:errorcluster, "Data out"=w133:T24)  [unwired: 8 out]
            n69 = call <resource>:"Reset layer template selection.vi"("error in (no error)"=w138, "Data in"=w133) -> ("error out"=w137:errorcluster, "Data out"=w132:T24)  [unwired: 1 in, 7 out]
          }
          event "Cancel": Value Change {
            n70 = event-data() -> ()  [unwired: 2 out]
            n71 = control-ref of="This VI"() -> (w144:refnum<vi>)
            n72 = call <resource>:"Verify Cancel.vi"("Calling VI"=w144) -> ("error out"=w147:errorcluster, "Close IE"=w146:bool)  [unwired: 9 in]
          }
          event Panel Close? {
            w150 = TRUE ("Discard?")
            n73 = event-data() -> ()  [unwired: 2 out]
            n74 = control-ref of="This VI"() -> (w149:refnum<vi>)
            n75 = call <resource>:"Verify Cancel.vi"("Calling VI"=w149) -> ("error out"=w152:errorcluster, "Close IE"=w151:bool)  [unwired: 9 in]
            n76 = event-data("Discard?"=w150) -> ()  [unwired: 1 in, 1 out]
          }
          event Mouse Up {
            # "Has check for anything changing"
            n77 = event-data() -> ()  [unwired: 2 out]
            n78 = Unbundle By Name(w162) -> ("Support.Action"=w160:T28, "Support.Mouse inside icon?"=w165:bool, "Support.Mouse Move Coords"=w161:T27)
            n79 = case shown="False" w165 {
              tunnel: w163 -> [w169 w180]
              tunnel: [w167 w180] -> w158
              tunnel: [w170 w179] -> w156
              tunnel: w162 -> [w171 w179]
              tunnel: w161 -> [w168 _]
              tunnel: w160 -> [w166 _]
              frame False {
                n80 = case shown="\"Move Selection\", \"Tool\"" w166 {
                  tunnel: w171 -> [w173 w178]
                  tunnel: [w173 w177] -> w170
                  tunnel: w169 -> [w172 w176]
                  tunnel: w168 -> [_ w175]
                  tunnel: [w172 w174] -> w167
                  frame "Default", Default {
                  }
                  frame "Move Selection", "Tool" {
                    n81 = call <resource>:"PictureControl_MouseUp.vi"("error in"=w176, "Coords"=w175, "Data in"=w178) -> ("error out"=w174:errorcluster, "Data out"=w177:T24)  [unwired: 4 in, 3 out]
                  }
                }
              }
              frame True {
              }
            }
            n82 = call <resource>:"Add Data to History.vi"("Check special fields? (F)"=TRUE, "Add to Undo?"=TRUE, "error in"=w158, "Data in"=w156) -> ("error out"=w157:errorcluster, "Data out"=w155:T24)  [unwired: 6 out]
          }
          event Key Down?; event type 5.0.x8000000b {
            n83 = event-data() -> ("Type"=w184:T31, "Char"=w181:i16, "VKey"=w188:T32, "PlatMods"=w183:T33)  [unwired: 1 out]
            n84 = call <resource>:"KeyDown.vi"("PlatMods"=w183, "Type"=w184, "error in (no error)"=w190, "VKey"=w188, "Char"=w181, "Data in"=w185) -> ("error out"=w189:errorcluster, "Discard?"=w187:bool, "Data out"=w182:T24)  [unwired: 3 out]
            n85 = event-data("Discard?"=w187) -> ()  [unwired: 1 in, 1 out]
          }
          event Key Up {
            n86 = event-data() -> ("PlatMods"=w192:T33)  [unwired: 1 out]
            n87 = call <resource>:"KeyUp.vi"("error in (no error)"=w194, "PlatMods"=w192, "Data in"=w193) -> ("error out"=w195:errorcluster, "Data out"=w191:T24)  [unwired: 7 out]
          }
          event Menu Selection (User); Menu Selection (App) {
            n88 = event-data() -> ("Type"=w208:T31, "ItemTag"=w209:string)  [unwired: 1 out]
            n89 = case shown="\"Text\"" w205 {
              tunnel: w207 -> [w211 w216]
              tunnel: w210 -> [w212 w215]
              tunnel: [w211 w214] -> w203
              tunnel: [w212 w213] -> w204
              frame Default {
              }
              frame "Text" {
                n90 = call <resource>:"Finalize Text.vi"("error in (no error)"=w216, "Data in"=w215) -> ("error out"=w214:errorcluster, "Data out"=w213:T24)  [unwired: 8 out]
              }
            }
            n91 = control-ref of="Clipboard"() -> (w196:refnum<vi>)
            n92 = case shown="\"Menu Selection (User)\"" w208 {
              tunnel: w209 -> [_ w225]
              tunnel: [w218 w224] -> w200
              tunnel: w203 -> [w218 w223]
              tunnel: w197 -> [_ w222]
              tunnel: w204 -> [w217 w221]
              tunnel: [w217 w220] -> w202
              tunnel: w196 -> [_ w219]
              frame Default {
              }
              frame "Menu Selection (User)" {
                n93 = call <resource>:"MenuSelection(User).vi"("User events"=w222, "Clipboard"=w219, "error in"=w223, "ItemTag"=w225, "Data in"=w221) -> ("error out"=w224:errorcluster, "Data out"=w220:T24)  [unwired: 5 out]
              }
            }
            n94 = call <resource>:"Add Data to History.vi"("Add to Undo?"=FALSE, "error in"=w200, "Data in"=w202) -> ("error out"=w199:errorcluster, "Data out"=w201:T24)  [unwired: 7 in]
          }
          event "Tab Control": Value Change {
            n95 = event-data() -> ("NewVal"=w237:T3)  [unwired: 1 out]
            n96 = case shown="\"Layers\", Default" w237 {
              tunnel: w236 -> [w241 w244 w246 w248]
              tunnel: [w240 w243 w247 w248] -> w235
              frame "Templates" {
                n97 = property on="Filter templates by keyword" class="Str"(error in=w241, "Key Focus"=TRUE) -> (error out=w240:errorcluster)  [unwired: 1 in, 1 out]
              }
              frame "Glyphs" {
                n98 = property on="Filter glyphs by keyword" class="Str"(error in=w244, "Key Focus"=TRUE) -> (error out=w243:errorcluster)  [unwired: 1 in, 1 out]
              }
              frame "Icon Text" {
                n99 = property on="Line 1 text" class="Str"(error in=w246, "Key Focus"=TRUE) -> (error out=w247:errorcluster)  [unwired: 1 in, 1 out]
              }
              frame "Layers", Default {
              }
            }
            n100 = call <resource>:"Finalize Text.vi"("error in (no error)"=w235, "Data in"=w232) -> ("error out"=w238:errorcluster, "Data out"=w231:T24)  [unwired: 8 out]
            n101 = call <resource>:"Finalize Movement.vi"("error in (no error)"=w238, "Data in"=w231) -> ("error out"=w230:errorcluster, "Data out"=w228:T24)  [unwired: 1 in, 7 out]
            n102 = call <resource>:"Escape.vi"("error in"=w230, "Data in"=w228) -> ("error out"=w229:errorcluster, "Data out"=w227:T24)  [unwired: 1 in, 7 out]
            n103 = call <resource>:"Reset layer template selection.vi"("error in (no error)"=w229, "Data in"=w227) -> ("error out"=w234:errorcluster, "Data out"=w226:T24)  [unwired: 1 in, 7 out]
          }
          event "Preview", "Terminals", "Preview2": Mouse Enter {
            n104 = event-data() -> ()  [unwired: 2 out]
            n105 = call <resource>:"SetCursor.vi"("error in (no error)"=w256, "Radio Buttons"=w254, "Data in"=w252) -> ("error out"=w255:errorcluster, "Data out"=w251:T24)  [unwired: 7 out]
            n106 = Bundle By Name(cluster=w251, "Support.Mouse inside icon?"=TRUE) -> (w250:T24)
          }
          event "Preview", "Terminals", "Preview2": Mouse Move {
            n107 = event-data() -> ("Coords"=w260:T27)  [unwired: 1 out]
            n108 = call <resource>:"CoordinatesCorrection.vi"("Coordinates In"=w260) -> ("Corrected Out"=w257:T27)  [unwired: 10 out]
            n109 = feedback-in #1(w257) -> ()
            n110 = feedback #1() -> (w259:T27)
            n111 = Not Equal?(x=w259, y=w257) -> (x != y?=w258:bool)
            n112 = case shown="True" w258 {
              tunnel: w266 -> [w268 w274]
              tunnel: [w268 w273] -> w265
              tunnel: w263 -> [_ w272]
              tunnel: w262 -> [w267 w271]
              tunnel: [w267 w270] -> w261
              tunnel: w257 -> [_ w269]
              frame False {
              }
              frame True {
                n113 = call <resource>:"MouseMove.vi"("Buffer"=w272, "error in"=w274, "Coords"=w269, "Data in"=w271) -> ("error out"=w273:errorcluster, "Data out"=w270:T24)  [unwired: 6 out]
              }
            }
          }
          event "Preview", "Preview2", "Terminals": Mouse Leave {
            n114 = event-data() -> ()  [unwired: 2 out]
            n115 = Bundle By Name(cluster=w275, "Support.Mouse inside icon?"=FALSE) -> (w277:T24)
          }
          event "Preview", "Terminals", "Preview2": Mouse Down {
            # "Left click"
            n116 = event-data() -> ("Button"=w281:u16, "Coords"=w294:T27)  [unwired: 1 out]
            n117 = Not Equal?(x=u16 1, y=w281) -> (x != y?=w279:bool)
            n118 = control-ref of="This VI"() -> (w290:refnum<vi>)
            n119 = call <resource>:"Defer_FP_Updates.vi"("Defer Panel Updates"=TRUE, "error in (no error)"=w296, "lv_icon.vi in"=w290) -> ("error out"=w286:errorcluster, "lv icon.vi out"=w288:refnum<vi>)  [unwired: 7 out]
            n120 = call <resource>:"Reset layer template selection.vi"("Force reset? (T)"=FALSE, "error in (no error)"=w286, "Data in"=w292) -> ("error out"=w285:errorcluster, "Data out"=w282:T24)  [unwired: 1 in, 6 out]
            n121 = call <resource>:"MouseDown.vi"("Flip colors?"=w279, "error in"=w285, "Coords"=w294, "Data in"=w282) -> ("error out"=w284:errorcluster, "Data out"=w291:T24)  [unwired: 1 in, 5 out]
            n122 = call <resource>:"Defer_FP_Updates.vi"("Defer Panel Updates"=FALSE, "error in (no error)"=w284, "lv_icon.vi in"=w288) -> ("error out"=w295:errorcluster)  [unwired: 8 out]
          }
          event "Preview", "Terminals", "Preview2": Mouse Up {
            n123 = event-data() -> ("Coords"=w301:T27)  [unwired: 1 out]
            n124 = call <resource>:"PictureControl_MouseUp.vi"("error in"=w302, "Coords"=w301, "Data in"=w298) -> ("error out"=w299:errorcluster, "Data out"=w297:T24)  [unwired: 4 in, 3 out]
          }
          event Value Change {
            n125 = event-data() -> ("NewVal"=w306:T20)  [unwired: 1 out]
            n126 = call <resource>:"Value Change_Tools.vi"("error in"=w307, "NewVal"=w306, "Data in"=w304) -> ("error out"=w305:errorcluster, "Data out"=w303:T24)  [unwired: 7 out]
          }
          event Mouse Down {
            n127 = event-data() -> ("Mods.Double Click"=w308:bool)  [unwired: 1 out]
            n128 = call <resource>:"Finalize Text.vi"("error in (no error)"=w314, "Data in"=w313) -> ("error out"=w316:errorcluster, "Data out"=w315:T24)  [unwired: 8 out]
            n129 = call <resource>:"Finalize Movement.vi"("error in (no error)"=w316, "Data in"=w315) -> ("error out"=w312:errorcluster, "Data out"=w311:T24)  [unwired: 1 in, 7 out]
            n130 = call <resource>:"Mouse Down.vi"("error in"=w312, "Double Click"=w308, "Data in"=w311) -> ("error out"=w309:errorcluster, "Data out"=w310:T24)  [unwired: 7 out]
            n131 = Bundle By Name(cluster=w310, "Support.Tool (old value)"=u32 111) -> (w318:T24)
          }
          event Mouse Down {
            n132 = event-data() -> ()  [unwired: 2 out]
            n133 = call <resource>:"Finalize Text.vi"("error in (no error)"=w326, "Data in"=w325) -> ("error out"=w327:errorcluster, "Data out"=w324:T24)  [unwired: 8 out]
            n134 = call <resource>:"Finalize Movement.vi"("error in (no error)"=w327, "Data in"=w324) -> ("error out"=w323:errorcluster, "Data out"=w321:T24)  [unwired: 1 in, 7 out]
            n135 = call <resource>:"Escape.vi"("error in"=w323, "Data in"=w321) -> ("error out"=w322:errorcluster, "Data out"=w320:T24)  [unwired: 1 in, 7 out]
          }
          event Value Change {
            n136 = event-data() -> ()  [unwired: 2 out]
            n137 = call <vilib>:"Check Color.vi"("Color in"="Fill Color") -> ("Color out"=w335:T19)  [unwired: 26 out]
            n138 = call <vilib>:"Check Color.vi"("Color in"="Line Color") -> ("Color out"=w336:T19)  [unwired: 26 out]
            n139 = Bundle By Name(cluster=w332, "Support.Fill Color"=w335, "Support.Edge Color"=w336) -> (w331:T24)
            n140 = call <resource>:"Escape.vi"("Reset cursor (T)"=FALSE ("Reset cursor? (T)"), "error in"=w333, "Data in"=w331) -> ("error out"=w334:errorcluster, "Data out"=w330:T24)  [unwired: 1 in, 6 out]
          }
          event Value Change {
            n141 = event-data() -> ()  [unwired: 2 out]
            n142 = call <resource>:"Finalize Text.vi"("error in (no error)"=w342, "Data in"=w344) -> ("error out"=w346:errorcluster, "Data out"=w345:T24)  [unwired: 8 out]
            n143 = local read "Line Color"() -> (w341:T19)
            n144 = local read "Fill Color"() -> (w351:T19)
            n145 = call <resource>:"Finalize Movement.vi"("error in (no error)"=w346, "Data in"=w345) -> ("error out"=w340:errorcluster, "Data out"=w343:T24)  [unwired: 1 in, 7 out]
            n146 = stacked-sequence {
              tunnel: w351 -> [w355]
              tunnel: [w354] -> w349
              tunnel: w341 -> [w353]
              tunnel: w340 -> [w352]
              frame #0 {
                n147 = local write "Fill Color"(w353) -> ()
                n148 = property on="Line Color" class="ColBox (strict)"(error in=w352, "Val(Sgnl)"=w355) -> (error out=w354:errorcluster)  [unwired: 1 in, 1 out]
              }
            }
            n149 = call <resource>:"Escape.vi"("error in"=w349, "Data in"=w343) -> ("error out"=w348:errorcluster, "Data out"=w347:T24)  [unwired: 1 in, 7 out]
          }
          event Value Change {
            n150 = event-data() -> ()  [unwired: 2 out]
            n151 = call <resource>:"Finalize Text.vi"("error in (no error)"=w365, "Data in"=w358) -> ("error out"=w364:errorcluster, "Data out"=w360:T24)  [unwired: 8 out]
            n152 = call <resource>:"Finalize Movement.vi"("error in (no error)"=w364, "Data in"=w360) -> ("error out"=w361:errorcluster, "Data out"=w357:T24)  [unwired: 1 in, 7 out]
            n153 = call <resource>:"RotateFlip.vi"("error in"=w361, "Rotate"="Clockwise Rotate", "Data in"=w357) -> ("error out"=w362:errorcluster, "Data out"=w356:T24)  [unwired: 2 in, 5 out]
            n154 = call <resource>:"Escape.vi"("error in"=w362, "Data in"=w356) -> ("error out"=w363:errorcluster, "Data out"=w359:T24)  [unwired: 1 in, 7 out]
          }
          event User Event {
            # "This is an initialization event for the templates"
            n155 = event-data() -> ("Templates"=w385:string)  [unwired: 1 out]
            n156 = Unbundle By Name(w370) -> ("Ref.TemplateLoadAnimation"=w369:refnum<vi>, "Ref.refreshTemplates"=w368:refnum<vi>)
            n157 = control-ref of="This VI"() -> (w380:refnum<vi>)
            n158 = call <resource>:"Defer_FP_Updates.vi"("Defer Panel Updates"=TRUE, "error in (no error)"=w383, "lv_icon.vi in"=w380) -> ("error out"=w378:errorcluster, "lv icon.vi out"=w377:refnum<vi>)  [unwired: 7 out]
            n159 = Unflatten From String(type=cluster{T6[], i32, bool} {[], 0, FALSE}, binary string=w385, error in (no error)=w378) -> (value=w376:cluster{T6[], i32, bool}, error out=w381:errorcluster)  [unwired: 3 out]
            n160 = call <resource>:"Process Template Graphics.vi"("error in (no error)"=w381, "Data"=w376, "Data in"=w370) -> ("error out"=w373:errorcluster, "Data out"=w375:T24)  [unwired: 7 out]
            n161 = call <resource>:"ChangeRefreshGraphicsState.vi"("error in (no error)"=w373, "refreshing?"=FALSE, "button ref"=w368, "animatedDecoration ref"=w369) -> ("error out"=w372:errorcluster)  [unwired: 7 in]
            n162 = call <resource>:"Defer_FP_Updates.vi"("error in (no error)"=w372, "lv_icon.vi in"=w377) -> ("error out"=w374:errorcluster)  [unwired: 1 in, 8 out]
          }
          event "Templates": Value Change {
            n163 = event-data() -> ("CtlRef"=w387:refnum<vi>, "NewVal"=w398:string)  [unwired: 1 out]
            n164 = control-ref of="This VI"() -> (w402:refnum<vi>)
            n165 = Unbundle By Name(w403) -> ("Class.Templates"=w390:refnum<class "FakedArray.lvclass">)
            n166 = call <resource>:"Defer_FP_Updates.vi"("Defer Panel Updates"=TRUE, "error in (no error)"=w400, "lv_icon.vi in"=w402) -> ("error out"=w392:errorcluster, "lv icon.vi out"=w397:refnum<vi>)  [unwired: 7 out]
            n167 = call-dynamic "SET_ScrollbarPosition.vi"("error in (no error)"=w392, "FakedArray.lvclass in"=w390) -> ("error out"=w394:errorcluster, "FakedArray.lvclass out"=w393:refnum<class "FakedArray.lvclass">)  [unwired: 1 in, 7 out]
            n168 = local write "Filter templates by keyword"("") -> ()
            n169 = call <resource>:"ResetColor.vi"("error in (no error)"=w394, "FakedArray in"=w393) -> ("error out"=w395:errorcluster, "FakedArray out"=w396:refnum<class "FakedArray.lvclass">)  [unwired: 8 out]
            n170 = call-dynamic "UpdateVisibleData.vi"("Templates tree"=w387, "error in (no error)"=w395, "Tag"=w398, "FakedArray in"=w396) -> ("error out"=w391:errorcluster, "FakedArray out"=w389:refnum<class "FakedArray.lvclass">)  [unwired: 1 in, 5 out]
            n171 = Bundle By Name(cluster=w403, "Class.Templates"=w389) -> (w388:T24)
            n172 = call <resource>:"Defer_FP_Updates.vi"("error in (no error)"=w391, "lv_icon.vi in"=w397) -> ("error out"=w399:errorcluster)  [unwired: 1 in, 8 out]
          }
          event "Templates": Mouse Down {
            n173 = event-data() -> ("CtlRef"=w408:refnum<vi>, "Coords"=w410:T27)  [unwired: 1 out]
            n174 = call <resource>:"Mouse Down_Tree.vi"("Tree"=w408, "error in (no error)"=w409, "Coords"=w410) -> ("error out"=w407:errorcluster)  [unwired: 8 out]
            n175 = call <resource>:"Escape.vi"("error in"=w407, "Data in"=w405) -> ("error out"=w406:errorcluster, "Data out"=w404:T24)  [unwired: 1 in, 7 out]
          }
          event Value Change {
            n176 = event-data() -> ("OldVal.Opacity"=w415:u8, "NewVal.Opacity"=w416:u8, "NewVal"=w420:T14)  [unwired: 1 out]
            n177 = Not Equal?(x=w415, y=w416) -> (x != y?=w414:bool)
            n178 = call <resource>:"Value Change_Top or Bottom Layer.vi"("Type"=enum16{"Template Layer", "Text Layer"}."Template Layer", "error in (no error)"=w422, "Data"=w420, "Data in"=w413) -> ("error out"=w418:errorcluster, "Data out"=w412:T24)  [unwired: 6 out]
            n179 = case shown="False" w414 {
              tunnel: w418 -> [w424 w428]
              tunnel: [w424 w427] -> w417
              tunnel: w412 -> [w423 w426]
              tunnel: [w423 w425] -> w411
              frame False {
              }
              frame True {
                n180 = call <resource>:"Reset layer template selection.vi"("error in (no error)"=w428, "Data in"=w426) -> ("error out"=w427:errorcluster, "Data out"=w425:T24)  [unwired: 1 in, 7 out]
              }
            }
          }
          event Mouse Down {
            n181 = event-data() -> ("CtlRef"=w434:refnum<vi>, "Button"=w430:u16)  [unwired: 1 out]
            n182 = case shown="1, 2" w430 {
              tunnel: w435 -> [w437 w444]
              tunnel: w434 -> [_ w448]
              tunnel: [w437 w442] -> w433
              tunnel: w431 -> [w436 w439]
              tunnel: [w436 w438] -> w429
              frame 0, Default {
              }
              frame 1, 2 {
                n183 = control-ref of="This VI"() -> (w447:refnum<vi>)
                n184 = call <resource>:"Defer_FP_Updates.vi"("Defer Panel Updates"=TRUE, "error in (no error)"=w444, "lv_icon.vi in"=w447) -> ("error out"=w445:errorcluster, "lv icon.vi out"=w440:refnum<vi>)  [unwired: 7 out]
                n185 = call <resource>:"Template_MouseDown.vi"("Add to Undo?"=TRUE, "error in"=w445, "CtlRef"=w448, "Data in"=w439) -> ("error out"=w443:errorcluster, "Data out"=w438:T24)  [unwired: 1 in, 5 out]
                n186 = call <resource>:"Defer_FP_Updates.vi"("error in (no error)"=w443, "lv_icon.vi in"=w440) -> ("error out"=w442:errorcluster)  [unwired: 1 in, 8 out]
              }
            }
          }
          event Value Change {
            n187 = event-data() -> ("NewVal"=w459:variant)  [unwired: 1 out]
            n188 = control-ref of="This VI"() -> (w456:refnum<vi>)
            n189 = call <resource>:"Defer_FP_Updates.vi"("Defer Panel Updates"=TRUE, "error in (no error)"=w457, "lv_icon.vi in"=w456) -> ("error out"=w458:errorcluster, "lv icon.vi out"=w451:refnum<vi>)  [unwired: 7 out]
            n190 = call <resource>:"Mouse Down_Templates.vi"("Tag"="Templates", "error in"=w458, "NewVal"=w459, "Data in"=w450) -> ("error out"=w453:errorcluster, "Data out"=w449:T24)  [unwired: 1 in, 5 out]
            n191 = call <resource>:"Defer_FP_Updates.vi"("error in (no error)"=w453, "lv_icon.vi in"=w451) -> ("error out"=w454:errorcluster)  [unwired: 1 in, 8 out]
          }
          event "Filter templates by keyword": Value Change {
            n192 = event-data() -> ("NewVal"=w479:string)  [unwired: 1 out]
            n193 = Unbundle By Name(w467) -> ("Ref.Templates tree"=w465:refnum<vi>, "Class.Templates"=w468:refnum<class "FakedArray.lvclass">)
            n194 = control-ref of="This VI"() -> (w478:refnum<vi>)
            n195 = call <resource>:"Defer_FP_Updates.vi"("Defer Panel Updates"=TRUE, "error in (no error)"=w476, "lv_icon.vi in"=w478) -> ("error out"=w470:errorcluster, "lv icon.vi out"=w475:refnum<vi>)  [unwired: 7 out]
            n196 = call-dynamic "SET_ScrollbarPosition.vi"("error in (no error)"=w470, "FakedArray.lvclass in"=w468) -> ("error out"=w471:errorcluster, "FakedArray.lvclass out"=w472:refnum<class "FakedArray.lvclass">)  [unwired: 1 in, 7 out]
            n197 = call <resource>:"ResetColor.vi"("error in (no error)"=w471, "FakedArray in"=w472) -> ("error out"=w473:errorcluster, "FakedArray out"=w474:refnum<class "FakedArray.lvclass">)  [unwired: 8 out]
            n198 = call-dynamic "UpdateVisibleData.vi"("Templates tree"=w465, "error in (no error)"=w473, "Keyword"=w479, "FakedArray in"=w474) -> ("error out"=w469:errorcluster, "FakedArray out"=w466:refnum<class "FakedArray.lvclass">)  [unwired: 1 in, 5 out]
            n199 = Bundle By Name(cluster=w467, "Class.Templates"=w466) -> (w461:T24)
            n200 = call <resource>:"Defer_FP_Updates.vi"("error in (no error)"=w469, "lv_icon.vi in"=w475) -> ("error out"=w463:errorcluster)  [unwired: 1 in, 8 out]
            n201 = call <resource>:"Add Data to History.vi"("Add to Undo?"=TRUE, "error in"=w463, "Data in"=w461) -> ("error out"=w462:errorcluster, "Data out"=w460:T24)  [unwired: 7 out]
          }
          event "Filter templates by keyword": Mouse Down {
            # "If a mouse down event should\nselect the entered text, enable this case"
            n202 = event-data() -> ("CtlRef"=w489:refnum<vi>)  [unwired: 1 out]
            n203 = disable-structure shown="Enabled" {
              disable-tunnel: w489 -> [w494 _]
              disable-tunnel: w488 -> [w492 w495]
              disable-tunnel: [w490 w495] -> w487
              frame Disabled {
                n204 = property class="Str"(reference=w494, error in=w492, "Text.Selection Start"=u32 0 ("Text.Selection:Start"), "Text.Selection End"=-1 ("Text.Selection:End")) -> (error out=w490:errorcluster)  [unwired: 1 out]
              }
              frame Enabled {
              }
            }
            n205 = call <resource>:"Finalize Text.vi"("error in (no error)"=w487, "Data in"=w485) -> ("error out"=w486:errorcluster, "Data out"=w484:T24)  [unwired: 8 out]
            n206 = call <resource>:"DeselectLayer.vi"("error in (no error)"=w486, "Data in"=w484) -> ("error out"=w483:errorcluster, "Data out"=w482:T24)  [unwired: 8 out]
            n207 = call <resource>:"Escape.vi"("error in"=w483, "Data in"=w482) -> ("error out"=w480:errorcluster, "Data out"=w481:T24)  [unwired: 1 in, 7 out]
          }
          event Value Change {
            n208 = event-data() -> ()  [unwired: 2 out]
            n209 = Unbundle By Name(w498) -> ("Ref.TemplateLoadAnimation"=w496:refnum<vi>, "Ref.refreshTemplates"=w497:refnum<vi>)
            n210 = call <resource>:"Launch Dynamically Load Graphics.vi"("User events"=w499, "Path"=Pathes."Icon Templates", "error in (no error)"=w501, "button ref"=w497, "animatedDecoration ref"=w496) -> ("error out"=w500:errorcluster)  [unwired: 1 in, 5 out]
          }
          event Mouse Down {
            n211 = event-data() -> ("CtlRef"=w507:refnum<vi>)  [unwired: 1 out]
            n212 = property class="CmbBox (strict)"(reference=w507, error in=w506, "Text.Selection Start"=u32 0 ("Text.Selection:Start"), "Text.Selection End"=u32 1000 ("Text.Selection:End")) -> (error out=w505:errorcluster)  [unwired: 1 out]
          }
          event Mouse Down {
            n213 = event-data() -> ()  [unwired: 2 out]
            n214 = call <resource>:"Escape.vi"("error in"=w510, "Data in"=w512) -> ("error out"=w509:errorcluster, "Data out"=w511:T24)  [unwired: 1 in, 7 out]
          }
          event Mouse Down {
            n215 = event-data() -> ()  [unwired: 2 out]
            n216 = call <resource>:"MouseDown_Body Text.vi"("error in"=w517, "Data in"=w514) -> ("error out"=w516:errorcluster, "Data out"=w513:T24)  [unwired: 8 out]
          }
          event Value Change {
            # "Body Text Value Change event is fired programmatically during initialization so first call of this event is guaranteed to be a case we do not want to update the undo/redo information."
            n217 = event-data() -> ("OldVal"=w526:T7, "NewVal"=w525:T7, "OldVal.Body Text Spec.Alignment"=w530:T9)  [unwired: 1 out]
            n218 = Unbundle By Name(w526) -> ("Body Text Spec.Font"=w524:T8)
            n219 = Unbundle By Name(w525) -> ("Body Text Spec.Font"=w523:T8)
            n220 = local read "Tab Control"() -> (w521:T3)
            n221 = Unbundle By Name(w525) -> ("Body Text Spec.Alignment"=w531:T9)
            n222 = First Call?() -> (First Call?: T/F=w538:bool)
            n223 = Equal?(x=w521, y=T3."Icon Text") -> (x = y?=w519:bool)
            n224 = Not(x=w538) -> (.not. x?=w537:bool)
            n225 = Not Equal?(x=w524, y=w523) -> (x != y?=w522:bool)
            n226 = call <resource>:"Value Change_Body Text.vi"("Layer Icon"="Icon Text", "Add to Undo?"=w537, "error in"=w539, "NewVal"=w525, "Data in"=w535) -> ("error out"=w533:errorcluster, "Data out"=w532:T24)  [unwired: 5 out]
            n227 = And(x=w519, y=w522) -> (x .and. y?=w518:bool)
            n228 = Not Equal?(x=w531, y=w530) -> (x != y?=w529:bool)
            n229 = case shown="False" w518 {
              frame False {
              }
              frame True {
                n230 = property on="Line 1 text" class="Str"("Key Focus"=TRUE) -> ()  [unwired: 2 in, 2 out]
              }
            }
            n231 = call <resource>:"Alignment Value Change.vi"("Set Focus?"=w529, "error in"=w533, "NewVal"=w531, "Data in"=w532) -> ("error out"=w527:errorcluster, "Data out"=w528:T24)  [unwired: 6 out]
          }
          event Value Change {
            n232 = event-data() -> ("OldVal.Opacity"=w546:u8, "NewVal.Opacity"=w545:u8, "NewVal"=w551:T14)  [unwired: 1 out]
            n233 = Not Equal?(x=w546, y=w545) -> (x != y?=w544:bool)
            n234 = call <resource>:"Value Change_Top or Bottom Layer.vi"("Type"=enum16{"Template Layer", "Text Layer"}."Text Layer", "error in (no error)"=w552, "Data"=w551, "Data in"=w543) -> ("error out"=w548:errorcluster, "Data out"=w542:T24)  [unwired: 6 out]
            n235 = case shown="True" w544 {
              tunnel: w548 -> [w554 w558]
              tunnel: [w554 w557] -> w547
              tunnel: w542 -> [w553 w556]
              tunnel: [w553 w555] -> w541
              frame False {
              }
              frame True {
                n236 = call <resource>:"Reset layer template selection.vi"("error in (no error)"=w558, "Data in"=w556) -> ("error out"=w557:errorcluster, "Data out"=w555:T24)  [unwired: 1 in, 7 out]
              }
            }
          }
          event Value Change {
            n237 = event-data() -> ("NewVal"=w569:variant)  [unwired: 1 out]
            n238 = control-ref of="This VI"() -> (w566:refnum<vi>)
            n239 = call <resource>:"Defer_FP_Updates.vi"("Defer Panel Updates"=TRUE, "error in (no error)"=w565, "lv_icon.vi in"=w566) -> ("error out"=w564:errorcluster, "lv icon.vi out"=w561:refnum<vi>)  [unwired: 7 out]
            n240 = Variant To Data(error in=w564, type=0, Variant=w569) -> (data=w568:i32, error out=w570:errorcluster)
            n241 = call <resource>:"UpdateLayerView_ScrollbarChanged.vi"("error in"=w570, "Scrollbar Position"=w568, "Data in"=w560) -> ("error out"=w563:errorcluster, "Data out"=w559:T24)  [unwired: 7 out]
            n242 = call <resource>:"Defer_FP_Updates.vi"("error in (no error)"=w563, "lv_icon.vi in"=w561) -> ("error out"=w562:errorcluster)  [unwired: 1 in, 8 out]
          }
          event Mouse Down {
            n243 = event-data() -> ("PlatMods.Shift"=w574:bool, "CtlRef"=w584:refnum<vi>, "PlatMods.Ctrl"=w583:bool)  [unwired: 1 out]
            n244 = control-ref of="This VI"() -> (w580:refnum<vi>)
            n245 = call <resource>:"Defer_FP_Updates.vi"("Defer Panel Updates"=TRUE, "error in (no error)"=w581, "lv_icon.vi in"=w580) -> ("error out"=w579:errorcluster, "lv icon.vi out"=w576:refnum<vi>)  [unwired: 7 out]
            n246 = call <resource>:"Mouse Down_User Layers.vi"("Shift"=w574, "error in"=w579, "Ctrl"=w583, "CtlRef"=w584, "Data in"=w573) -> ("error out"=w578:errorcluster, "Data out"=w572:T24)  [unwired: 5 out]
            n247 = call <resource>:"Defer_FP_Updates.vi"("error in (no error)"=w578, "lv_icon.vi in"=w576) -> ("error out"=w577:errorcluster)  [unwired: 1 in, 8 out]
          }
          event Mouse Down {
            n248 = event-data() -> ("Button"=w587:u16)  [unwired: 1 out]
            n249 = case shown="1" w587 {
              tunnel: w589 -> [w591 w595]
              tunnel: [w591 w594] -> w588
              tunnel: w586 -> [w590 w593]
              tunnel: [w590 w592] -> w585
              frame 0, Default {
              }
              frame 1 {
                # "Left click"
                n250 = call <resource>:"Reset layer template selection.vi"("error in (no error)"=w595, "Data in"=w593) -> ("error out"=w594:errorcluster, "Data out"=w592:T24)  [unwired: 1 in, 7 out]
              }
            }
          }
          event Value Change {
            # "We do not use the dynamic registerd event for Layer Clust.Value Change\nbecause it would be a huge effort to lock the front panel until this\nevent case has been completed."
            n251 = event-data() -> ("OldVal.Visibility?"=w597:bool, "CtlRef"=w611:refnum<vi>, "OldVal.LayerName"=w596:string)  [unwired: 1 out]
            n252 = control-ref of="This VI"() -> (w608:refnum<vi>)
            n253 = call <resource>:"Defer_FP_Updates.vi"("Defer Panel Updates"=TRUE, "error in (no error)"=w607, "lv_icon.vi in"=w608) -> ("error out"=w606:errorcluster, "lv icon.vi out"=w603:refnum<vi>)  [unwired: 7 out]
            n254 = call <resource>:"LayerCluster_ValueChange.vi"("Old Visibility?"=w597, "error in"=w606, "Old name"=w596, "CtlRef"=w611, "Data in"=w599) -> ("error out"=w605:errorcluster, "Data out"=w600:T24)  [unwired: 1 in, 4 out]
            n255 = call <resource>:"Defer_FP_Updates.vi"("Defer Panel Updates"=FALSE, "error in (no error)"=w605, "lv_icon.vi in"=w603) -> ("error out"=w602:errorcluster)  [unwired: 8 out]
            n256 = call <resource>:"Reset layer template selection.vi"("error in (no error)"=w602, "Data in"=w600) -> ("error out"=w601:errorcluster, "Data out"=w598:T24)  [unwired: 1 in, 7 out]
          }
          event Value Change {
            n257 = event-data() -> ()  [unwired: 2 out]
            n258 = control-ref of="This VI"() -> (w622:refnum<vi>)
            n259 = call <resource>:"Defer_FP_Updates.vi"("Defer Panel Updates"=TRUE, "error in (no error)"=w621, "lv_icon.vi in"=w622) -> ("error out"=w619:errorcluster, "lv icon.vi out"=w618:refnum<vi>)  [unwired: 7 out]
            n260 = call <resource>:"Add new Layer.vi"("error in"=w619, "Data in"=w623) -> ("error out"=w614:errorcluster, "Data out"=w616:T24)  [unwired: 8 out]
            n261 = call <resource>:"ViewLayer.vi"("Add to Undo?"=TRUE, "error in (no error)"=w614, "Data in"=w616) -> ("error out"=w613:errorcluster, "Data out"=w615:T24)  [unwired: 1 in, 6 out]
            n262 = call <resource>:"Defer_FP_Updates.vi"("error in (no error)"=w613, "lv_icon.vi in"=w618) -> ("error out"=w617:errorcluster)  [unwired: 1 in, 8 out]
          }
          event Mouse Leave; Mouse Up {
            n263 = event-data() -> ()  [unwired: 2 out]
            n264 = call <resource>:"Add Data to History.vi"("Add to Undo?"=TRUE, "error in"=w627, "Data in"=w624) -> ("error out"=w626:errorcluster, "Data out"=w625:T24)  [unwired: 7 out]
          }
          event Value Change {
            n265 = event-data() -> ()  [unwired: 2 out]
            n266 = control-ref of="This VI"() -> (w639:refnum<vi>)
            n267 = Unbundle By Name(w645) -> ("Class.Icon"=w644:refnum<class "Icon.lvclass">)
            n268 = call <resource>:"Defer_FP_Updates.vi"("Defer Panel Updates"=TRUE, "error in (no error)"=w638, "lv_icon.vi in"=w639) -> ("error out"=w637:errorcluster, "lv icon.vi out"=w636:refnum<vi>)  [unwired: 7 out]
            n269 = call-dynamic "GET_All User Layers.vi"("error in (no error)"=w637, "Icon.lvclass in"=w644) -> ("error out"=w651:errorcluster, "User Layer"=w647:refnum<class "Layer.lvclass">[], "Icon.lvclass out"=w646:refnum<class "Icon.lvclass">)  [unwired: 7 out]
            n270 = call <resource>:"Delete Selected Layers.vi"("error in"=w651, "All Layers in"=w647, "Data in"=w645) -> ("error out"=w650:errorcluster, "All Layers out"=w648:refnum<class "Layer.lvclass">[], "Data out"=w642:T24)
            n271 = call-dynamic "SET_UserLayers.vi"("error in (no error)"=w650, "Layers"=w648, "Icon.lvclass in"=w646) -> ("error out"=w649:errorcluster, "Icon.lvclass out"=w643:refnum<class "Icon.lvclass">)  [unwired: 7 in]
            n272 = Bundle By Name(cluster=w642, "Class.Icon"=w643) -> (w641:T24)
            n273 = call <resource>:"Reset layer template selection.vi"("error in (no error)"=w649, "Data in"=w641) -> ("error out"=w630:errorcluster, "Data out"=w632:T24)  [unwired: 1 in, 7 out]
            n274 = call <resource>:"ViewLayer.vi"("Add to Undo?"=TRUE, "error in (no error)"=w630, "Data in"=w632) -> ("error out"=w629:errorcluster, "Data out"=w631:T24)  [unwired: 2 in, 5 out]
            n275 = call <resource>:"Defer_FP_Updates.vi"("error in (no error)"=w629, "lv_icon.vi in"=w636) -> ("error out"=w635:errorcluster)  [unwired: 1 in, 8 out]
          }
          event Value Change {
            n276 = event-data() -> ()  [unwired: 2 out]
            n277 = control-ref of="This VI"() -> (w662:refnum<vi>)
            n278 = call <resource>:"Defer_FP_Updates.vi"("Defer Panel Updates"=TRUE, "error in (no error)"=w661, "lv_icon.vi in"=w662) -> ("error out"=w660:errorcluster, "lv icon.vi out"=w659:refnum<vi>)  [unwired: 7 out]
            n279 = call <resource>:"MoveLayers.vi"("error in"=w660, "Arrow Up"="Move Up", "Data in"=w656) -> ("error out"=w652:errorcluster, "Data out"=w655:T24)  [unwired: 7 out]
            n280 = stacked-sequence {
              tunnel: [w665] -> w653
              tunnel: w652 -> [w665]
              frame #0 {
                w666 = FALSE ("Arrow Down")
                n281 = local write "Move Down"(w666) -> ()
                n282 = local write "Move Up"(w666) -> ()
              }
            }
            n283 = call <resource>:"Defer_FP_Updates.vi"("Defer Panel Updates"=FALSE, "error in (no error)"=w653, "lv_icon.vi in"=w659) -> ("error out"=w658:errorcluster)  [unwired: 8 out]
          }
          event User Event {
            # "This is an initialization event for the glyphs."
            n284 = event-data() -> ("Glyphs"=w681:string)  [unwired: 1 out]
            n285 = Unbundle By Name(w669) -> ("Ref.GlyphLoadAnimation"=w668:refnum<vi>, "Ref.refreshGlyphs"=w667:refnum<vi>)
            n286 = Unflatten From String(type=T30[] [], binary string=w681, error in (no error)=w679) -> (value=w676:T30[], error out=w678:errorcluster)  [unwired: 3 out]
            n287 = call <resource>:"Populate Graphics.vi"("error in"=w678, "Glyphs []"=w676, "Data in"=w669) -> ("error out"=w677:errorcluster, "Data out"=w673:T24)  [unwired: 7 out]
            n288 = call <resource>:"Write Glyphs to  File.vi"("File Name"="Glyphs.bin", "Path"=Pathes."Glyphs", "error in (no error)"=w677, "Graphics []"=w676) -> ("error out"=w672:errorcluster)  [unwired: 7 out]
            n289 = call <resource>:"ChangeRefreshGraphicsState.vi"("error in (no error)"=w672, "refreshing?"=FALSE, "button ref"=w667, "animatedDecoration ref"=w668) -> ("error out"=w671:errorcluster)  [unwired: 7 in]
          }
          event "Glyphs": Mouse Down {
            n290 = event-data() -> ("CtlRef"=w683:refnum<vi>, "Coords"=w688:T27)  [unwired: 1 out]
            n291 = local write "Filter glyphs by keyword"("") -> ()
            n292 = call <resource>:"Mouse Down_Tree.vi"("Tree"=w683, "error in (no error)"=w689, "Coords"=w688) -> ("error out"=w687:errorcluster)  [unwired: 8 out]
            n293 = call <resource>:"Escape.vi"("error in"=w687, "Data in"=w685) -> ("error out"=w686:errorcluster, "Data out"=w684:T24)  [unwired: 1 in, 7 out]
          }
          event "Glyphs": Value Change {
            n294 = event-data() -> ("NewVal"=w697:string)  [unwired: 1 out]
            n295 = Unbundle By Name(w693) -> ("Class.Glyph"=w694:refnum<class "Glyph.lvclass">, "Ref.DNL_Glyphs []"=w690:refnum<vi>)
            n296 = call <resource>:"FilterGlyphs.vi"("error in (no error)"=w695, "DNL_Glyphs []"=w690, "Tag"=w697, "Glyph in"=w694) -> ("error out"=w696:errorcluster, "Glyph out"=w692:refnum<class "Glyph.lvclass">)  [unwired: 6 out]
            n297 = Bundle By Name(cluster=w693, "Class.Glyph"=w692) -> (w691:T24)
          }
          event "Filter glyphs by keyword": Mouse Down {
            # "If a mouse down event should\nselect the entered text, enable this case"
            n298 = event-data() -> ("CtlRef"=w706:refnum<vi>)  [unwired: 1 out]
            n299 = disable-structure shown="Disabled" {
              disable-tunnel: w707 -> [w710 w713]
              disable-tunnel: w706 -> [w709 _]
              disable-tunnel: [w708 w713] -> w705
              frame Disabled {
                n300 = property class="Str"(reference=w709, error in=w710, "Text.Selection Start"=u32 0 ("Text.Selection:Start"), "Text.Selection End"=-1 ("Text.Selection:End")) -> (error out=w708:errorcluster)  [unwired: 1 out]
              }
              frame Enabled {
              }
            }
            n301 = call <resource>:"Finalize Text.vi"("error in (no error)"=w705, "Data in"=w703) -> ("error out"=w704:errorcluster, "Data out"=w702:T24)  [unwired: 8 out]
            n302 = call <resource>:"DeselectLayer.vi"("error in (no error)"=w704, "Data in"=w702) -> ("error out"=w701:errorcluster, "Data out"=w700:T24)  [unwired: 8 out]
            n303 = call <resource>:"Escape.vi"("error in"=w701, "Data in"=w700) -> ("error out"=w698:errorcluster, "Data out"=w699:T24)  [unwired: 1 in, 7 out]
          }
          event "Filter glyphs by keyword": Value Change {
            n304 = event-data() -> ("NewVal"=w727:string)  [unwired: 1 out]
            n305 = Unbundle By Name(w722) -> ("Class.Glyph"=w723:refnum<class "Glyph.lvclass">, "Ref.DNL_Glyphs []"=w720:refnum<vi>, "Ref.Glyphs tree"=w719:refnum<vi>)
            n306 = First Call?() -> (First Call?: T/F=w725:bool)
            n307 = Not(x=w725) -> (.not. x?=w726:bool)
            n308 = call <resource>:"SearchGlyphs.vi"("Glyphs tree"=w719, "DNL_Glyphs []"=w720, "Reset position? (F)"=w726, "error in (no error)"=w724, "Keyword"=w727, "Glyph in"=w723) -> ("error out"=w718:errorcluster, "Glyph out"=w721:refnum<class "Glyph.lvclass">)  [unwired: 4 out]
            n309 = Bundle By Name(cluster=w722, "Class.Glyph"=w721) -> (w715:T24)
            n310 = call <resource>:"Add Data to History.vi"("Add to Undo?"=TRUE, "error in"=w718, "Data in"=w715) -> ("error out"=w717:errorcluster, "Data out"=w716:T24)  [unwired: 7 out]
          }
          event "Glyphs []": Mouse Down {
            n311 = event-data() -> ("Button"=w736:u16, "Mods.Double Click"=w737:bool, "CtlRef"=w739:refnum<vi>, "Coords"=w740:T27)  [unwired: 1 out]
            n312 = case shown="1" w736 {
              tunnel: w740 -> [_ w749]
              tunnel: w739 -> [_ w748]
              tunnel: [w742 w747] -> w733
              tunnel: w738 -> [w742 w746]
              tunnel: w737 -> [_ w745]
              tunnel: w731 -> [w741 w744]
              tunnel: [w741 w743] -> w729
              frame 0, Default {
              }
              frame 1 {
                # "Left click"
                n313 = call <resource>:"Mouse Down_Glyphs.vi"("Double Click"=w745, "Coords"=w749, "error in"=w746, "CtlRef"=w748, "Data in"=w744) -> ("error out"=w747:errorcluster, "Data out"=w743:T24)  [unwired: 1 in, 4 out]
              }
            }
            n314 = call <resource>:"Reset layer template selection.vi"("error in (no error)"=w733, "Data in"=w729) -> ("error out"=w732:errorcluster, "Data out"=w730:T24)  [unwired: 1 in, 7 out]
            n315 = call <resource>:"Update glyph path string.vi"("error in (no error)"=w732, "Data in"=w730) -> ("error out"=w734:errorcluster, "Data out"=w728:T24)  [unwired: 1 in, 7 out]
          }
          event Value Change {
            n316 = event-data() -> ()  [unwired: 2 out]
            n317 = Unbundle By Name(w752) -> ("Ref.GlyphLoadAnimation"=w750:refnum<vi>, "Ref.refreshGlyphs"=w751:refnum<vi>)
            n318 = call <resource>:"Launch Dynamically Load Graphics.vi"("User events"=w753, "Path"=Pathes."Glyphs", "error in (no error)"=w755, "button ref"=w751, "animatedDecoration ref"=w750) -> ("error out"=w754:errorcluster)  [unwired: 1 in, 5 out]
          }
          event "Help": Value Change {
            n319 = event-data() -> ()  [unwired: 2 out]
            n320 = control-ref of="This VI"() -> (w759:refnum<vi>)
            n321 = property class="VI"(reference=w759) -> (error out=w757:errorcluster, "Help.URL"=w758:string)  [unwired: 1 in, 1 out]
            n322 = call <resource>:"IE_Open Help Link.vi"("error in (no error)"=w757, "Help.URL"=w758) -> ()  [unwired: 9 in, 1 out]
          }
          event "Glyphs", "Templates": Item Close; "Glyphs", "Templates": event #0x1e {
            n323 = event-data() -> ("CtlRef"=w762:refnum<vi>)  [unwired: 1 out]
            n324 = call <resource>:"DealWithScrollbars.vi"("error in (no error)"=w764, "Tree"=w762) -> ("error out"=w763:errorcluster)  [unwired: 9 in]
          }
        }
        n325 = case shown="True" w110 {
          tunnel: [_ w126] -> w113
          tunnel: w112 -> [w123 w129]
          tunnel: [w123 w128] -> w111
          tunnel: "Tools" -> [_ w127]
          tunnel: w121 -> [w122 w125]
          tunnel: [w122 w124] -> w120
          frame False {
          }
          frame True {
            n326 = call <resource>:"DrawIcon.vi"("Tools"=w127, "error in (no error)"=w129, "Data in"=w125) -> ("error out"=w128:errorcluster, "Icon"=w126:picture, "Data out"=w124:T24, "RGB"=→"RGB":string, "XYL"=→"XYZ":string)  [unwired: 2 in, 2 out]
            "Icon" <- w126
            "Preview" <- w126
          }
        }
        n327 = Or(x=w112, y=w117) -> (x .or. y?=w116:bool)
      }
      n328 = call <resource>:"Buffer for lossless tracking.vi"("Ref Cluster"=w91, "User events"=w79, "error in (no error)"=w95, "Buffer"=w94) -> ()  [unwired: 8 out]
      n329 = call <resource>:"Extract LV Icon Data.vi"("error in (no error)"=w85, "LabVIEW Icon in (original)"=w83, "Data in"=w87) -> ("error out"=w84:errorcluster, "LabVIEW Icon out"=w86:string, "Data out"=w82:T24)  [unwired: 6 in]
      n330 = call <vilib>:"Get Image Data.vi"("Pic In"=w102) -> ("image data out"=w90:T2)  [unwired: 2 in, 8 out]
      n331 = call <vilib>:"Get Image Data.vi"("depth (24)"=1 ("depth"), "Pic In"=w102) -> ("image data out"=w100:T2)  [unwired: 2 in, 7 out]
      n332 = call <resource>:"SetCursor.vi"("Radio Buttons"=Tools."Select", "Data in"=w82) -> ("Data out"=w81:T24)  [unwired: 8 in, 1 out]
      n333 = Unbundle By Name(w84) -> ("code"=w103:i32)
      n334 = flat-sequence {
        tunnel: w106 -> [w766]
        tunnel: w104 -> [w774]
        tunnel: w84 -> [w773]
        tunnel: w79 -> [w771]
        tunnel: w81 -> [w767]
        frame #0 {
          n335 = Unbundle By Name(w771) -> ("Global stop?"=w770:refnum<user-event>, "Templates"=w769:refnum<user-event>, "Glyphs"=w768:refnum<user-event>)
          n336 = call <resource>:"Write INI Tokens and VI Tags.vi"("error in"=w773, "Global Data in"=w767) -> ()  [unwired: 1 in, 9 out]
          n337 = Unregister For Events(event registration refnum=w766) -> ()  [unwired: 1 in, 1 out]
          n338 = Release Notifier(notifier=w774, force destroy? (F)=TRUE) -> ()  [unwired: 1 in, 3 out]
          n339 = call <resource>:"Call Keep IE in Memory.vi"() -> ()  [unwired: 1 out]
          n340 = Generate User Event(user event=w770, event data cluster=TRUE) -> ()  [unwired: 2 in, 2 out]
          n341 = Destroy User Event(user event=w769) -> ()  [unwired: 1 in, 1 out]
          n342 = Destroy User Event(user event=w768) -> ()  [unwired: 1 in, 1 out]
        }
        frame #1 {
          n343 = invoke class="VI" method="FP.Close"() -> ()  [unwired: 3 in, 3 out]
        }
      }
      n344 = call-dynamic "GET_Notifier.vi"("error in (no error)"=w88, "Ants.lvclass in"=w92) -> ("error out"=w98:errorcluster, "Notifier"=w104:refnum<notifier>, "Ants.lvclass out"=w99:refnum<class "Ants.lvclass">)  [unwired: 7 out]
      n345 = call <resource>:"RunningAnts.vi"("error in (no error)"=w98, "Ants in"=w99) -> ()  [unwired: 10 out]
    }
    frame Error {
      n346 = Unbundle By Name(w777) -> ("code"=w778:i32)
      n347 = call <vilib>:"Simple Error Handler.vi"("error in (no error)"=w777) -> ()  [unwired: 4 in, 5 out]
    }
  }
  "BW icon out" <- w54
  "Error code out" <- w58
  "Color icon out" <- w36
  "LabVIEW Icon out" <- w33
